vi "Lab Panel V2.4.vi"() -> ()   [LabVIEW 2013]
uses:
  <vilib>/Platform/TimedLoop/XDataNode/timing_clust.ctl
  <vilib>/Platform/TimedLoop/XDataNode/nitl_modes.ctl
  <vilib>/Platform/TimedLoop/XDataNode/wakeup.ctl
  <vilib>/platform/TimedLoop/XDataNode/XDataNode.xnode
  <vilib>/Platform/TimedLoop/XDataNode/XDNodeRunTimeDep.lvlib
panel:
  out "TEMP update":bool
  out "AI update":bool
  in  "stop":bool
  in  "Tab Control 2":T1(tab)
  out "LAB05-2 (SIG)":T2 {"PF" format="%.2f"; "AMPS" format="%.1f"}
  out "LAB05-1 (SIG)":T2 {"PF" format="%.2f"; "AMPS" format="%.1f"}
  out "LAB04-2 (SIG)":T2 {"PF" format="%.2f"; "AMPS" format="%.1f"}
  out "LAB04-1 (SIG)":T2 {"PF" format="%.2f"; "AMPS" format="%.1f"}
  out "LAB03-2 (SIG)":T2 {"PF" format="%.2f"; "AMPS" format="%.1f"}
  out "LAB03-1 (SIG)":T2 {"PF" format="%.2f"; "AMPS" format="%.1f"}
  out "LAB02-2 (SIG)":T2 {"PF" format="%.2f"; "AMPS" format="%.1f"}
  in  "LAB01-1RUN":bool
  in  "LAB05-1 (O/I)":bool
  in  "LAB05-2 (O/I)":bool
  in  "LAB04-1 (O/I)":bool
  in  "LAB04-2 (O/I)":bool
  in  "LAB02-1 (O/I)":bool
  in  "LAB02-2 (O/I)":bool
  in  "LAB01-2 (O/I)":bool
  in  "LAB01-1 (O/I)":bool
  in  "LAB03-1 (O/I)":bool
  in  "LAB05-2 RUN":bool
  in  "LAB05-1 RUN":bool
  in  "LAB04-2 RUN":bool
  in  "LAB04-1 RUN":bool
  in  "LAB03-2 RUN":bool
  in  "LAB03-1 RUN":bool
  in  "LAB02-2 RUN":bool
  in  "LAB02-1 RUN":bool
  in  "LAB01-2 RUN":bool
  in  "LAB05-2 SELECT":T3(radio)
  in  "LAB05-1 SELECT":T3(radio)
  in  "LAB04-2 SELECT":T3(radio)
  in  "LAB04-1 SELECT":T3(radio)
  in  "LAB03-2 SELECT":T3(radio)
  in  "LAB03-1 SELECT":T3(radio)
  in  "LAB02-2 SELECT":T3(radio)
  in  "LAB02-1 SELECT":T3(radio)
  in  "LAB01-2 SELECT":T3(radio)
  in  "LAB01-1 SELECT":T3(radio)
  in  "LAB03-2 (O/I)":bool
  out "LAB01-1 (SIG)":T2 {"PF" format="%.2f"; "AMPS" format="%.1f"}
  out "LAB01-2 (SIG)":T2 {"PF" format="%.2f"; "AMPS" format="%.1f"}
  out "LAB02-1 (SIG)":T2 {"PF" format="%.2f"; "AMPS" format="%.1f"}
  out "LAB05-2 (RESULT)":bool
  out "LAB05-1 (RESULT)":bool
  out "LAB04-2 (RESULT)":bool
  out "LAB04-1 (RESULT)":bool
  out "LAB03-2 (RESULT)":bool
  out "LAB03-1 (RESULT)":bool
  out "LAB02-2 (RESULT)":bool
  out "LAB02-1 (RESULT)":bool
  out "LAB01-2 (RESULT)":bool
  out "LAB01-1 (RESULT)":bool
  in  "LAB05 (SETTINGS 1)":T4={"1 Name"="", "1 Description"="", "1 (CYCLES)"=1.0, "1 (T-RISE mins)"=1.0, "1 (T-RISE deg C)"=1.0, "2 Name"="", "2 Description"="", "2 (CYCLES)"=1.0, "2 (T-RISE mins)"=1.0, "2 (T-RISE deg C)"=1.0} {"2 (T-RISE deg C)" min=1.0 max=100.0 step=1.0 format="%#.0f"; "2 (T-RISE mins)" min=0.0 max=1000.0 step=10.0 format="%#.0f"; "2 (CYCLES)" min=0.0 max=100000.0 step=10.0; "1 (T-RISE deg C)" min=1.0 max=100.0 step=1.0 format="%#.0f"; "1 (T-RISE mins)" min=0.0 max=1000.0 step=10.0 format="%#.0f"; "1 (CYCLES)" min=0.0 max=100000.0 step=10.0}
  in  "LAB04 (SETTINGS 1)":T4={"1 Name"="", "1 Description"="", "1 (CYCLES)"=1.0, "1 (T-RISE mins)"=1.0, "1 (T-RISE deg C)"=1.0, "2 Name"="", "2 Description"="", "2 (CYCLES)"=1.0, "2 (T-RISE mins)"=1.0, "2 (T-RISE deg C)"=1.0} {"2 (T-RISE deg C)" min=1.0 max=100.0 step=1.0 format="%#.0f"; "2 (T-RISE mins)" min=0.0 max=1000.0 step=10.0 format="%#.0f"; "2 (CYCLES)" min=0.0 max=100000.0 step=10.0; "1 (T-RISE deg C)" min=1.0 max=100.0 step=1.0 format="%#.0f"; "1 (T-RISE mins)" min=0.0 max=1000.0 step=10.0 format="%#.0f"; "1 (CYCLES)" min=0.0 max=100000.0 step=10.0}
  in  "LAB03 (SETTINGS 1)":T4={"1 Name"="", "1 Description"="", "1 (CYCLES)"=1.0, "1 (T-RISE mins)"=1.0, "1 (T-RISE deg C)"=1.0, "2 Name"="", "2 Description"="", "2 (CYCLES)"=1.0, "2 (T-RISE mins)"=1.0, "2 (T-RISE deg C)"=1.0} {"2 (T-RISE deg C)" min=1.0 max=100.0 step=1.0 format="%#.0f"; "2 (T-RISE mins)" min=0.0 max=1000.0 step=10.0 format="%#.0f"; "2 (CYCLES)" min=0.0 max=100000.0 step=10.0; "1 (T-RISE deg C)" min=1.0 max=100.0 step=1.0 format="%#.0f"; "1 (T-RISE mins)" min=0.0 max=1000.0 step=10.0 format="%#.0f"; "1 (CYCLES)" min=0.0 max=100000.0 step=10.0}
  out "LAB05 (DISP 1)":T5 {"2 (T-RISE min)" format="%#.0f"; "2 (CYCLE)" format="%#.0f"; "1 (T-RISE min)" format="%#.0f"; "1 (CYCLE)" format="%#.0f"}
  out "LAB04 (DISP 1)":T5 {"2 (T-RISE min)" format="%#.0f"; "2 (CYCLE)" format="%#.0f"; "1 (T-RISE min)" format="%#.0f"; "1 (CYCLE)" format="%#.0f"}
  out "LAB03 (DISP 1)":T5 {"2 (T-RISE min)" format="%#.0f"; "2 (CYCLE)" format="%#.0f"; "1 (T-RISE min)" format="%#.0f"; "1 (CYCLE)" format="%#.0f"}
  out "LAB02 (DISP 1)":T5 {"2 (T-RISE min)" format="%#.0f"; "2 (CYCLE)" format="%#.0f"; "1 (T-RISE min)" format="%#.0f"; "1 (CYCLE)" format="%#.0f"}
  in  "LAB02 (SETTINGS 1)":T4={"1 Name"="", "1 Description"="", "1 (CYCLES)"=1.0, "1 (T-RISE mins)"=1.0, "1 (T-RISE deg C)"=1.0, "2 Name"="", "2 Description"="", "2 (CYCLES)"=1.0, "2 (T-RISE mins)"=1.0, "2 (T-RISE deg C)"=1.0} {"2 (T-RISE deg C)" min=1.0 max=100.0 step=1.0 format="%#.0f"; "2 (T-RISE mins)" min=0.0 max=1000.0 step=10.0 format="%#.0f"; "2 (CYCLES)" min=0.0 max=100000.0 step=10.0; "1 (T-RISE deg C)" min=1.0 max=100.0 step=1.0 format="%#.0f"; "1 (T-RISE mins)" min=0.0 max=1000.0 step=10.0 format="%#.0f"; "1 (CYCLES)" min=0.0 max=100000.0 step=10.0}
  out "LAB01 (DISP 1)":T5 {"2 (T-RISE min)" format="%#.0f"; "2 (CYCLE)" format="%#.0f"; "1 (T-RISE min)" format="%.2f"; "1 (CYCLE)" format="%#.0f"}
  in  "LAB01 (SETTINGS 1)":T4={"1 Name"="", "1 Description"="", "1 (CYCLES)"=1.0, "1 (T-RISE mins)"=1.0, "1 (T-RISE deg C)"=1.0, "2 Name"="", "2 Description"="", "2 (CYCLES)"=1.0, "2 (T-RISE mins)"=1.0, "2 (T-RISE deg C)"=1.0} {"2 (T-RISE deg C)" min=1.0 max=100.0 step=1.0 format="%#.0f"; "2 (T-RISE mins)" min=0.0 max=1000.0 step=10.0 format="%#.0f"; "2 (CYCLES)" min=0.0 max=100000.0 step=10.0; "1 (T-RISE deg C)" min=1.0 max=100.0 step=1.0 format="%#.0f"; "1 (T-RISE mins)" min=1.0 max=1000.0 step=10.0 format="%#.0f"; "1 (CYCLES)" min=1.0 max=100000.0 step=10.0}
  out "LAB05 (TEMP START)":T6
  out "LAB04 (TEMP START)":T6
  out "LAB03 (TEMP START)":T6
  out "LAB02 (TEMP START)":T6
  out "LAB01 (TEMP START)":T6
  in  "JIG ON TIME (S)":dbl=1.0 min=1.0 max=10.0 step=0.5 format="%.1g"
  in  "JIG OFF TIME (S)":dbl=2.0 min=2.0 max=10.0 step=0.5 format="%.1g"
  out "LAB01-1 (JIG)":bool
  out "LAB01-2 (JIG)":bool
  out "LAB02-1 (JIG)":bool
  out "LAB02-2 (JIG)":bool
  out "LAB03-1 (JIG)":bool
  out "LAB03-2 (JIG)":bool
  out "LAB04-1 (JIG)":bool
  out "LAB04-2 (JIG)":bool
  out "LAB05-1 (JIG)":bool
  out "LAB05-2 (JIG)":bool
  out "LAB01 (CAL)":T7 {"2 (TN) cal" min=0.0 step=0.01 format="%.2f"; "2 (TL) cal" min=0.0 step=0.01 format="%.2f"; "2 (PF) cal" min=0.0 step=0.01 format="%.2f"; "2 (V) cal" min=0.0 step=0.01 format="%.2f"; "2 (A) cal" min=0.0 step=0.01 format="%.2f"; "1 (TN) cal" min=0.0 step=0.01 format="%.2f"; "1 (TL) cal" min=0.0 step=0.01 format="%.2f"; "1 (PF) cal" min=0.0 step=0.01 format="%.2f"; "1 (V) cal" min=0.0 step=0.01 format="%.2f"; "1  (A) cal" min=0.0 step=0.01 format="%.2f"}
  out "LAB03 (CAL)":T7 {"2 (TN) cal" min=0.0 step=0.01 format="%.2f"; "2 (TL) cal" min=0.0 step=0.01 format="%.2f"; "2 (PF) cal" min=0.0 step=0.01 format="%.2f"; "2 (V) cal" min=0.0 step=0.01 format="%.2f"; "2 (A) cal" min=0.0 step=0.01 format="%.2f"; "1 (TN) cal" min=0.0 step=0.01 format="%.2f"; "1 (TL) cal" min=0.0 step=0.01 format="%.2f"; "1 (PF) cal" min=0.0 step=0.01 format="%.2f"; "1 (V) cal" min=0.0 step=0.01 format="%.2f"; "1  (A) cal" min=0.0 step=0.01 format="%.2f"}
  out "LAB02 (CAL)":T8 {"2 (TN) cal" min=0.0 step=0.01 format="%.2f"; "2 (TL) cal" min=0.0 step=0.01 format="%.2f"; "2 (PF) cal" min=0.0 step=0.01 format="%.2f"; "2 (V) cal" min=0.0 step=0.01 format="%.2f"; "2 (A) cal" min=0.0 step=0.01 format="%.2f"; "1 (TN) cal" min=0.0 step=0.01 format="%.2f"; "1 (TL) cal" min=0.0 step=0.01 format="%.2f"; "1 (PF) cal" min=0.0 step=0.01 format="%.2f"; "1 (V) cal" min=0.0 step=0.01 format="%.2f"; "1 (A) cal" min=0.0 step=0.01 format="%.2f"}
  out "LAB05 (CAL)":T7 {"2 (TN) cal" min=0.0 step=0.01 format="%.2f"; "2 (TL) cal" min=0.0 step=0.01 format="%.2f"; "2 (PF) cal" min=0.0 step=0.01 format="%.2f"; "2 (V) cal" min=0.0 step=0.01 format="%.2f"; "2 (A) cal" min=0.0 step=0.01 format="%.2f"; "1 (TN) cal" min=0.0 step=0.01 format="%.2f"; "1 (TL) cal" min=0.0 step=0.01 format="%.2f"; "1 (PF) cal" min=0.0 step=0.01 format="%.2f"; "1 (V) cal" min=0.0 step=0.01 format="%.2f"; "1  (A) cal" min=0.0 step=0.01 format="%.2f"}
  out "LAB04 (CAL)":T7 {"2 (TN) cal" min=0.0 step=0.01 format="%.2f"; "2 (TL) cal" min=0.0 step=0.01 format="%.2f"; "2 (PF) cal" min=0.0 step=0.01 format="%.2f"; "2 (V) cal" min=0.0 step=0.01 format="%.2f"; "2 (A) cal" min=0.0 step=0.01 format="%.2f"; "1 (TN) cal" min=0.0 step=0.01 format="%.2f"; "1 (TL) cal" min=0.0 step=0.01 format="%.2f"; "1 (PF) cal" min=0.0 step=0.01 format="%.2f"; "1 (V) cal" min=0.0 step=0.01 format="%.2f"; "1  (A) cal" min=0.0 step=0.01 format="%.2f"}
  out "calibration file error out":errorcluster
  in  "CALIBRATE":bool
  in  "Tab Control":T9(tab)
  out "LAB01-2 (GRAPH)":dynamicdata(graph)
  out "LAB01-1 (GRAPH)":dynamicdata(graph)
  out "LAB02-2 (GRAPH)":dynamicdata(graph)
  out "LAB02-1 (GRAPH)":dynamicdata(graph)
  out "LAB03-2 (GRAPH)":dynamicdata(graph)
  out "LAB03-1 (GRAPH)":dynamicdata(graph)
  out "LAB04-2 (GRAPH)":dynamicdata(graph)
  out "LAB04-1 (GRAPH)":dynamicdata(graph)
  out "LAB05-2 (GRAPH)":dynamicdata(graph)
  out "LAB05-1 (GRAPH)":dynamicdata(graph)
  out "LAB05 TEMP":T10
  out "LAB04 TEMP":T10
  out "LAB02 TEMP":T10
  out "LAB01 TEMP":T10
  out "LAB03 TEMP":T10
  out "Analog Error Array":errorcluster[](array[cluster])
  out "AI loop time":dbl format="%.6g"
  out "loops":dbl
  in  "loop  delay(mS)":dbl
  out "on loops":dbl
  out "off loops":dbl
  out "jig cycle":dbl
  out "LAB01-1 (TDMS)":refnum<k34>
  out "LAB01-2 (TDMS)":refnum<k34>
  out "data file error":errorcluster
  # "LAB01"
  # "LAB02"
  # "LAB05"
  # "LAB03"
  # "LAB04"
  # "LAB01"
  # "LAB02"
  # "LAB03"
  # "LAB04"
  # "LAB05"
  # "JIG SET"
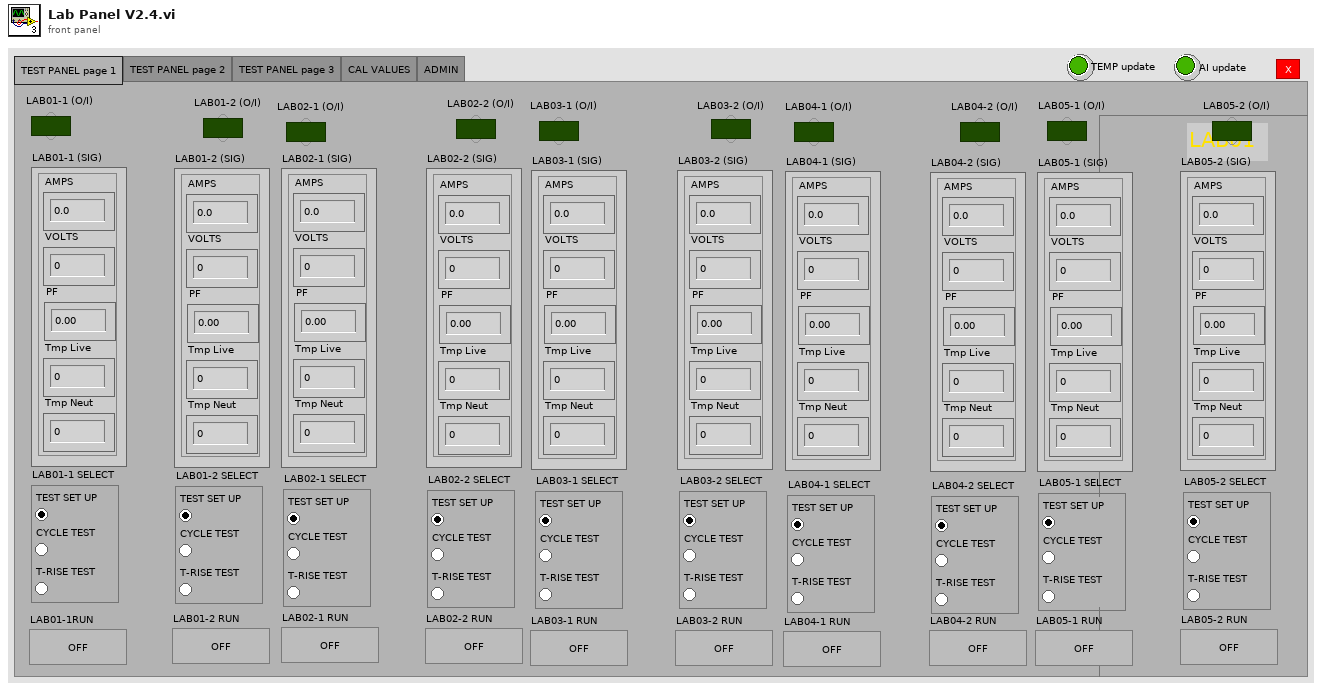
[diagram p1: front panel]
types:
  T1 = enum32{"TEST PANEL page 1", "TEST PANEL page 2", "TEST PANEL page 3", "CAL VALUES", "ADMIN"}
  T2 = cluster{"AMPS":dbl, "VOLTS":dbl, "PF":dbl, "Tmp Live":dbl, "Tmp Neut":dbl}
  T3 = enum32{"TEST SET UP", "CYCLE TEST", "T-RISE TEST"}
  T4 = cluster{"1 Name":string, "1 Description":string, "1 (CYCLES)":dbl, "1 (T-RISE mins)":dbl, "1 (T-RISE deg C)":dbl, "2 Name":string, "2 Description":string, "2 (CYCLES)":dbl, "2 (T-RISE mins)":dbl, "2 (T-RISE deg C)":dbl}
  T5 = cluster{"1 (CYCLE)":dbl, "1 (T-RISE min)":dbl, "1 (STATUS)":string, "2 (CYCLE)":dbl, "2 (T-RISE min)":dbl, "2 (STATUS)":string}
  T6 = cluster{"1 (TL)":dbl, "1 (TN)":dbl, "2 (TL)":dbl, "2 (TN)":dbl}
  T7 = cluster{"1  (A) cal":dbl, "1 (V) cal":dbl, "1 (PF) cal":dbl, "1 (TL) cal":dbl, "1 (TN) cal":dbl, "2 (A) cal":dbl, "2 (V) cal":dbl, "2 (PF) cal":dbl, "2 (TL) cal":dbl, "2 (TN) cal":dbl}
  T8 = cluster{"1 (A) cal":dbl, "1 (V) cal":dbl, "1 (PF) cal":dbl, "1 (TL) cal":dbl, "1 (TN) cal":dbl, "2 (A) cal":dbl, "2 (V) cal":dbl, "2 (PF) cal":dbl, "2 (TL) cal":dbl, "2 (TN) cal":dbl}
  T9 = enum32{"LAB01", "LAB02", "LAB03", "LAB04", "LAB05", "TEMPERATURE", "ERROR"}
  T10 = cluster{"T1 Live":dbl, "T1 Neut":dbl, "T2 Live":dbl, "T2 Neut":dbl, "ID":dbl, "ER":dbl}
  T11 = typedef "XDNodeRunTimeDep.lvlib/timing_clust.ctl" = cluster{"Expected End [f-1]":u64, "Actual End [f-1]":u64, "Finished Late? [f-1]":bool, "Expected End [i-1]":u64, "Actual End [i-1]":u64, "Finished Late? [i-1]":bool, "Expected Start [i]":u64, "Actual Start [i]":u64, "Expected Start [f]":u64, "Actual Start [f]":u64, "Source Name":string, "Structure Name":string, "Period":i64, "Deadline":i64, "Offset":i64, "Start":i64, "Priority":i32, "Timeout":i32, "Mode":T12, "Wakeup Reason":T13, "Error":errorcluster, "Source Type":string, "Secondary Source Type":string, "Global End Time":u64, "Global Start Time":u64, "Frame Duration":u64, "Iteration Duration":u64, "Assigned CPU":i32, "I/O Scan Engine Mode":u32}
  T12 = typedef "XDNodeRunTimeDep.lvlib/nitl_modes.ctl" = enum32{"No Change", "Process missed periods, maintain original phase", "Discard missed periods, maintain original phase", "Process missed periods, ignore original phase", "Discard missed periods, ignore original phase"}
  T13 = typedef "XDNodeRunTimeDep.lvlib/wakeup.ctl" = enum32{"Normal", "Aborted", "Asynchronous wakeup", "Timing source error", "Timed loop error", "Timeout"}
  T14 = enum16{"open", "open or create", "create or replace", "create", "open (read-only)"}
  T15 = cluster{"T1":dbl, "T2":dbl, "T3":dbl, "T4":dbl, "ID":dbl, "ER":dbl}
  T16 = cluster{"LAB01-1 (A)":dbl, "LAB01-1 (V)":dbl, "LAB01-1 (PF)":dbl, "LAB01-2 (A)":dbl, "LAB01-2 (V)":dbl, "LAB01-2 (PF)":dbl}
  T17 = cluster{"LAB02-1 (A)":dbl, "LAB02-1 (V)":dbl, "LAB02-1 (PF)":dbl, "LAB02-2 (A)":dbl, "LAB02-2 (V)":dbl, "LAB02-2 (PF)":dbl}
  T18 = cluster{"LAB03-1 (A)":dbl, "LAB03-1 (V)":dbl, "LAB03-1 (PF)":dbl, "LAB03-2 (A)":dbl, "LAB03-2 (V)":dbl, "LAB03-2 (PF)":dbl}
  T19 = cluster{"LAB04-1 (A)":dbl, "LAB04-1 (V)":dbl, "LAB04-1 (PF)":dbl, "LAB04-2 (A)":dbl, "LAB04-2 (V)":dbl, "LAB04-2 (PF)":dbl}
  T20 = cluster{"LAB05-1 (A)":dbl, "LAB05-1 (V)":dbl, "LAB05-1 (PF)":dbl, "LAB05-2 (A)":dbl, "LAB05-2 (V)":dbl, "LAB05-2 (PF)":dbl}
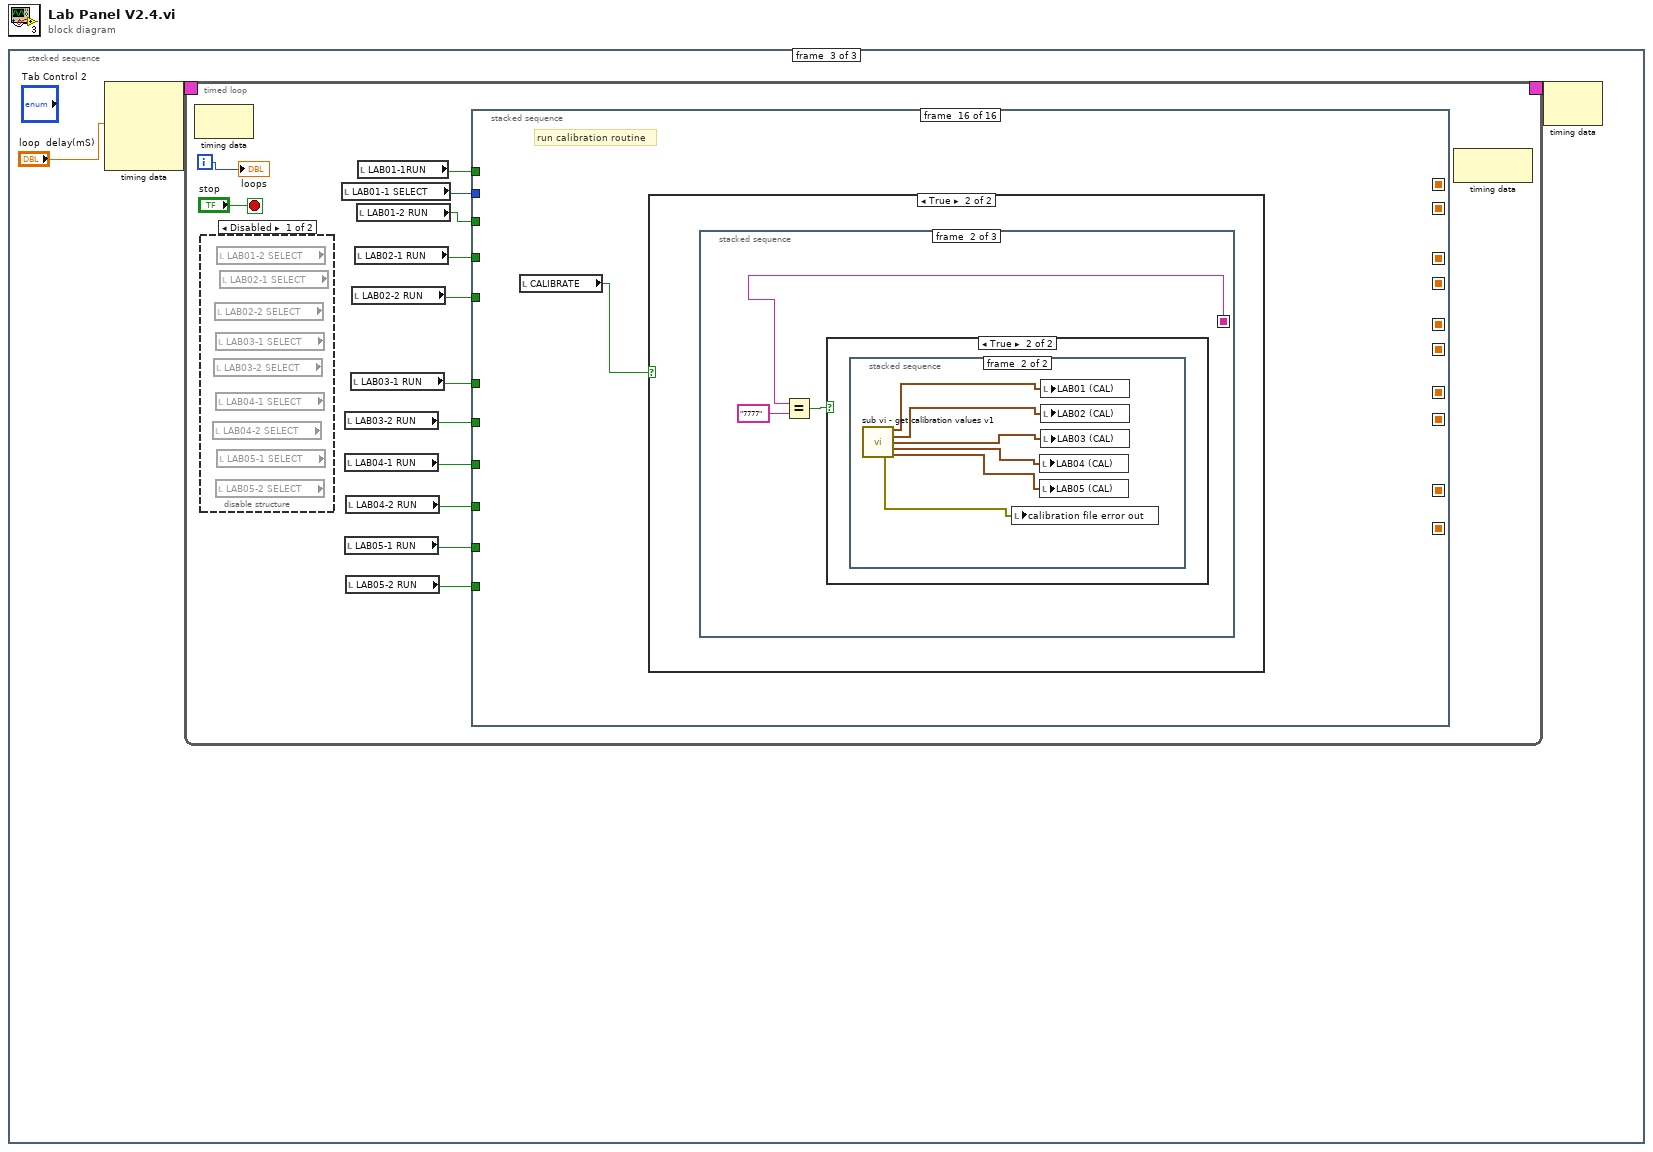
[diagram p0: block diagram]
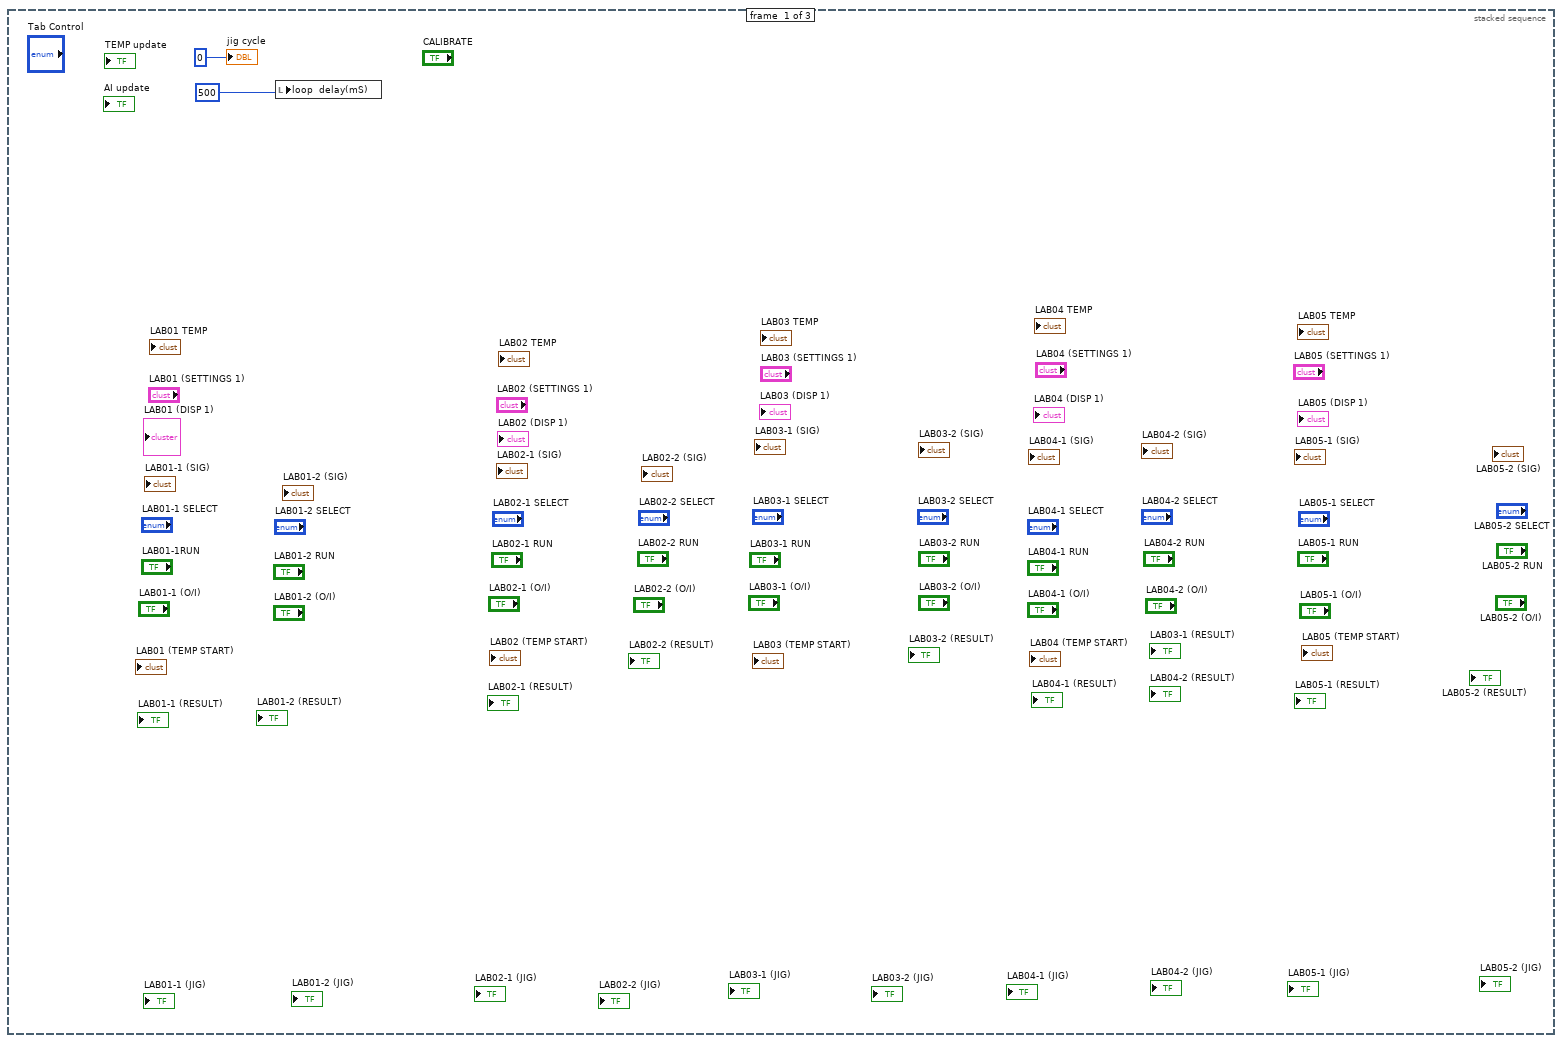
[diagram p2: hidden frame]
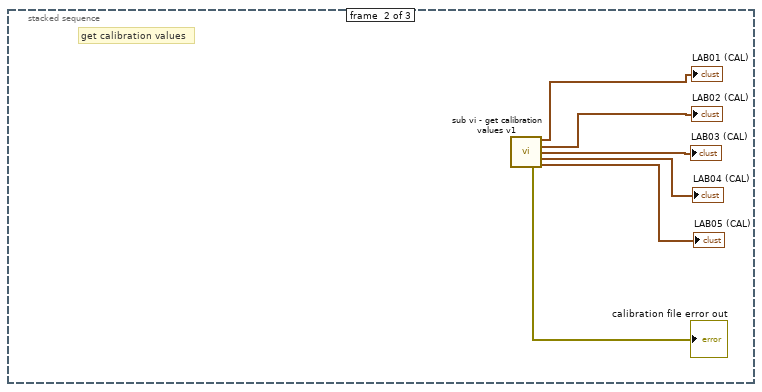
[diagram p3: hidden frame]
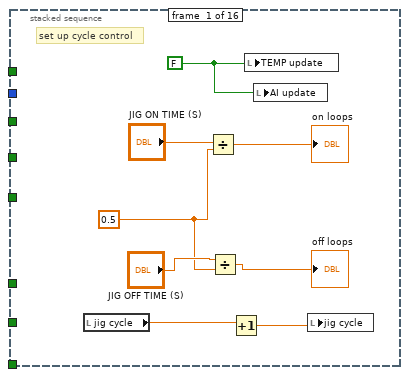
[diagram p5: hidden frame]
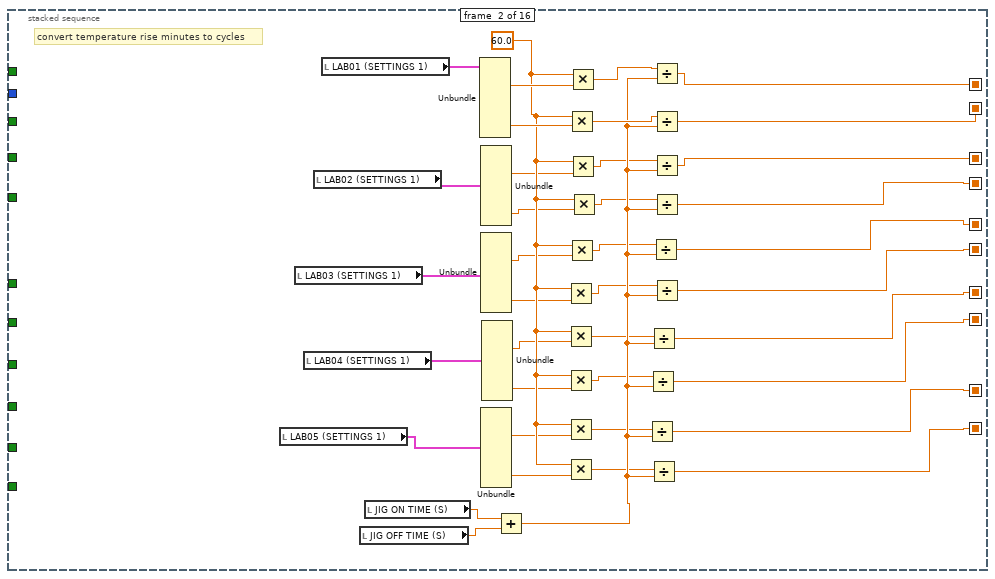
[diagram p6: hidden frame]
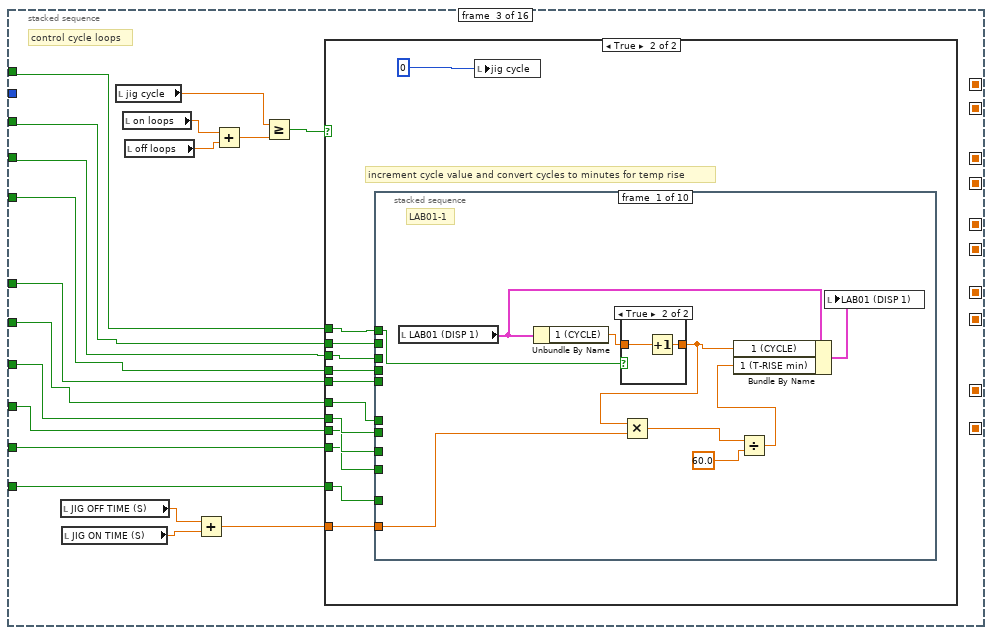
[diagram p7: hidden frame]
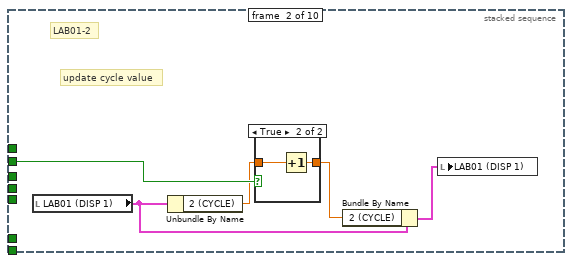
[diagram p10: hidden frame]
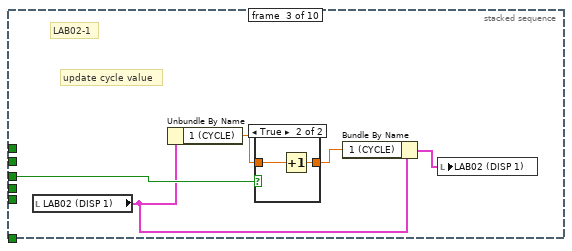
[diagram p12: hidden frame]
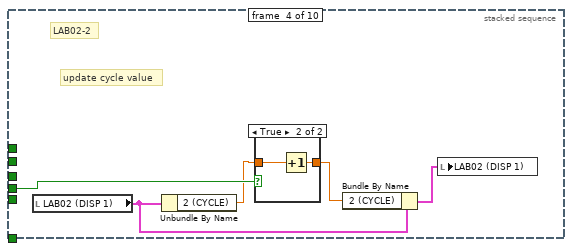
[diagram p14: hidden frame]
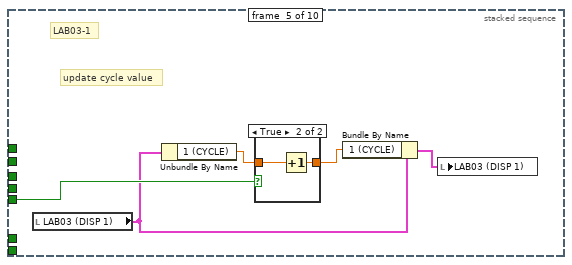
[diagram p16: hidden frame]
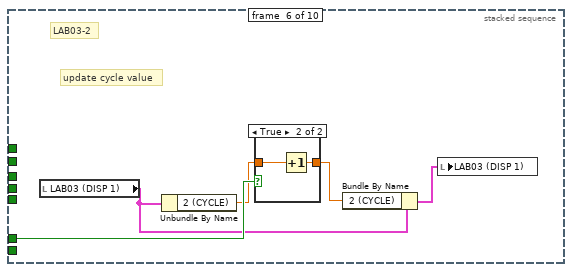
[diagram p18: hidden frame]
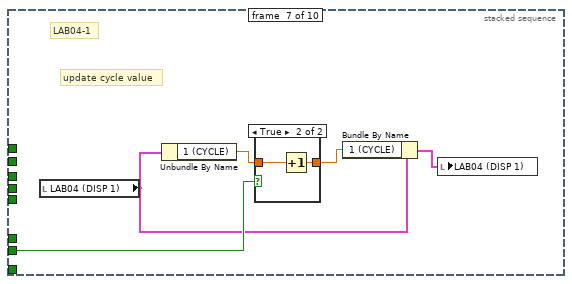
[diagram p20: hidden frame]
diagram:
  n1 = stacked-sequence {
    frame #0 {
      n2 = local write "loop  delay(mS)"(500) -> ()
      "jig cycle" <- 0
    }
    frame #1 {
      # "get calibration values"
      n3 = call "sub vi - get calibration values v1.vi"() -> ("LAB01 (CAL)"=→"LAB01 (CAL)":T7, "LAB02 (CAL)"=→"LAB02 (CAL)":T8, "LAB03 (CAL)"=→"LAB03 (CAL)":T7, "LAB04 (CAL)"=→"LAB04 (CAL)":T7, "calibration file error out"=→"calibration file error out":errorcluster, "LAB05 (CAL)"=→"LAB05 (CAL)":T7)  [unwired: 10 in]
    }
    frame #2 {
      n4 = node-c288("loop  delay(mS)") -> (w11:T11)  [unwired: 3 in]
      n5 = timed-loop {
        timing: w11 -> [_]
        timing-out: [_] -> w10
        i -> [w24]
        stop <- "stop" stop-if-true
        n6 = node-c288() -> ()  [unwired: 1 in, 1 out]
        n7 = disable-structure shown="Disabled" {
          frame Disabled {
            n8 = local read "LAB04-2 SELECT"() -> ()  [unwired: 1 out]
            n9 = local read "LAB03-2 SELECT"() -> ()  [unwired: 1 out]
            n10 = local read "LAB02-2 SELECT"() -> ()  [unwired: 1 out]
            n11 = local read "LAB03-1 SELECT"() -> ()  [unwired: 1 out]
            n12 = local read "LAB04-1 SELECT"() -> ()  [unwired: 1 out]
            n13 = local read "LAB05-2 SELECT"() -> ()  [unwired: 1 out]
            n14 = local read "LAB01-2 SELECT"() -> ()  [unwired: 1 out]
            n15 = local read "LAB05-1 SELECT"() -> ()  [unwired: 1 out]
            n16 = local read "LAB02-1 SELECT"() -> ()  [unwired: 1 out]
          }
          frame Enabled {
          }
        }
        n17 = local read "LAB01-1 SELECT"() -> (w12:T3)
        n18 = local read "LAB03-2 RUN"() -> (w17:bool)
        n19 = local read "LAB04-1 RUN"() -> (w16:bool)
        n20 = local read "LAB05-1 RUN"() -> (w14:bool)
        n21 = local read "LAB04-2 RUN"() -> (w15:bool)
        n22 = local read "LAB05-2 RUN"() -> (w13:bool)
        n23 = local read "LAB03-1 RUN"() -> (w18:bool)
        n24 = local read "LAB02-2 RUN"() -> (w19:bool)
        n25 = local read "LAB02-1 RUN"() -> (w20:bool)
        n26 = local read "LAB01-2 RUN"() -> (w21:bool)
        n27 = local read "LAB01-1RUN"() -> (w22:bool)
        n28 = stacked-sequence {
          seq-local: [_ w70 _ _ _ _ _ _ _ _ _ _ _ _ _ _] -> [_ _ _ _ w235 _ _ _ _ _ _ _ _ _ _ _]
          seq-local: [_ w69 _ _ _ _ _ _ _ _ _ _ _ _ _ _] -> [_ _ _ _ _ _ _ _ _ _ _ _ _ _ _ _]
          seq-local: [_ w42 _ _ _ _ _ _ _ _ _ _ _ _ _ _] -> [_ _ _ _ _ _ _ _ _ _ _ _ _ _ _ _]
          seq-local: [_ w41 _ _ _ _ _ _ _ _ _ _ _ _ _ _] -> [_ _ _ _ _ _ _ _ _ _ _ _ _ _ _ _]
          seq-local: [_ w40 _ _ _ _ _ _ _ _ _ _ _ _ _ _] -> [_ _ _ _ _ _ _ _ _ _ _ _ _ _ _ _]
          seq-local: [_ w39 _ _ _ _ _ _ _ _ _ _ _ _ _ _] -> [_ _ _ _ _ _ _ _ _ _ _ _ _ _ _ _]
          seq-local: [_ w38 _ _ _ _ _ _ _ _ _ _ _ _ _ _] -> [_ _ _ _ _ _ _ _ _ _ _ _ _ _ _ _]
          seq-local: [_ w37 _ _ _ _ _ _ _ _ _ _ _ _ _ _] -> [_ _ _ _ _ _ _ _ _ _ _ _ _ _ _ _]
          seq-local: [_ w36 _ _ _ _ _ _ _ _ _ _ _ _ _ _] -> [_ _ _ _ _ _ _ _ _ _ _ _ _ _ _ _]
          seq-local: [_ w35 _ _ _ _ _ _ _ _ _ _ _ _ _ _] -> [_ _ _ _ _ _ _ _ _ _ _ _ _ _ _ _]
          tunnel: w22 -> [_ _ w87 w198 w246 w283 w346 _ _ _ _ _ w809 w865 w924 _]
          tunnel: w21 -> [_ _ w86 w197 w245 w282 _ _ _ _ _ _ _ _ _ _]
          tunnel: w20 -> [_ _ w85 w196 w244 w281 _ _ _ _ _ _ _ _ _ _]
          tunnel: w19 -> [_ _ w84 w195 w243 w280 _ _ _ _ _ _ _ _ _ _]
          tunnel: w18 -> [_ _ w83 w194 w242 w279 _ _ _ _ _ _ _ _ _ _]
          tunnel: w17 -> [_ _ w82 w193 w241 w278 _ _ _ _ _ _ _ _ _ _]
          tunnel: w16 -> [_ _ w81 w192 w240 w277 _ _ _ _ _ _ _ _ _ _]
          tunnel: w15 -> [_ _ w80 w191 w239 w276 _ _ _ _ _ _ _ _ _ _]
          tunnel: w14 -> [_ _ w79 w190 w238 w275 _ _ _ _ _ _ _ _ _ _]
          tunnel: w13 -> [_ _ w78 w189 w237 w274 _ _ _ _ _ _ _ _ _ _]
          tunnel: w12 -> [_ _ _ w188 w236 _ w347 _ _ _ _ _ _ w867 w925 _]
          frame #0 {
            w27 = FALSE
            w32 = 0.5
            # "set up cycle control"
            n29 = local read "jig cycle"() -> (w31:dbl)
            n30 = Divide(x="JIG ON TIME (S)", y=w32) -> (x/y=→"on loops":dbl)
            n31 = Divide(x="JIG OFF TIME (S)", y=w32) -> (x/y=→"off loops":dbl)
            n32 = Increment(x=w31) -> (x+1=w30:dbl)
            n33 = local write "TEMP update"(w27) -> ()
            n34 = local write "AI update"(w27) -> ()
            n35 = local write "jig cycle"(w30) -> ()
          }
          frame #1 {
            w60 = 60.0
            # "convert temperature rise minutes to cycles"
            n36 = local read "LAB05 (SETTINGS 1)"() -> (w61:T4)
            n37 = local read "LAB03 (SETTINGS 1)"() -> (w63:T4)
            n38 = local read "LAB04 (SETTINGS 1)"() -> (w62:T4)
            n39 = local read "LAB02 (SETTINGS 1)"() -> (w64:T4)
            n40 = local read "LAB01 (SETTINGS 1)"() -> (w73:T4)
            n41 = local read "JIG OFF TIME (S)"() -> (w71:dbl)
            n42 = local read "JIG ON TIME (S)"() -> (w72:dbl)
            n43 = Unbundle(w73) -> ("1 (T-RISE mins)"=w68:dbl, "2 (T-RISE mins)"=w67:dbl)  [unwired: 8 out]
            n44 = Unbundle(w64) -> ("1 (T-RISE mins)"=w59:dbl, "2 (T-RISE mins)"=w58:dbl)  [unwired: 8 out]
            n45 = Unbundle(w63) -> ("1 (T-RISE mins)"=w57:dbl, "2 (T-RISE mins)"=w56:dbl)  [unwired: 8 out]
            n46 = Unbundle(w61) -> ("1 (T-RISE mins)"=w53:dbl, "2 (T-RISE mins)"=w52:dbl)  [unwired: 8 out]
            n47 = Unbundle(w62) -> ("1 (T-RISE mins)"=w55:dbl, "2 (T-RISE mins)"=w54:dbl)  [unwired: 8 out]
            n48 = Add(x=w72, y=w71) -> (x+y=w51:dbl)
            n49 = Multiply(x=w60, y=w56) -> (x*y=w47:dbl)
            n50 = Multiply(x=w60, y=w55) -> (x*y=w46:dbl)
            n51 = Multiply(x=w60, y=w54) -> (x*y=w45:dbl)
            n52 = Multiply(x=w60, y=w53) -> (x*y=w44:dbl)
            n53 = Multiply(x=w60, y=w52) -> (x*y=w43:dbl)
            n54 = Multiply(x=w60, y=w67) -> (x*y=w65:dbl)
            n55 = Multiply(x=w60, y=w57) -> (x*y=w48:dbl)
            n56 = Multiply(x=w60, y=w68) -> (x*y=w66:dbl)
            n57 = Multiply(x=w60, y=w59) -> (x*y=w50:dbl)
            n58 = Multiply(x=w60, y=w58) -> (x*y=w49:dbl)
            n59 = Divide(x=w44, y=w51) -> (x/y=w36:dbl)
            n60 = Divide(x=w45, y=w51) -> (x/y=w37:dbl)
            n61 = Divide(x=w46, y=w51) -> (x/y=w38:dbl)
            n62 = Divide(x=w43, y=w51) -> (x/y=w35:dbl)
            n63 = Divide(x=w48, y=w51) -> (x/y=w40:dbl)
            n64 = Divide(x=w66, y=w51) -> (x/y=w70:dbl)
            n65 = Divide(x=w65, y=w51) -> (x/y=w69:dbl)
            n66 = Divide(x=w50, y=w51) -> (x/y=w42:dbl)
            n67 = Divide(x=w49, y=w51) -> (x/y=w41:dbl)
            n68 = Divide(x=w47, y=w51) -> (x/y=w39:dbl)
          }
          frame #2 {
            # "control cycle loops"
            n69 = local read "JIG OFF TIME (S)"() -> (w76:dbl)
            n70 = local read "JIG ON TIME (S)"() -> (w75:dbl)
            n71 = local read "jig cycle"() -> (w89:dbl)
            n72 = local read "on loops"() -> (w91:dbl)
            n73 = local read "off loops"() -> (w90:dbl)
            n74 = Add(x=w76, y=w75) -> (x+y=w74:dbl)
            n75 = Add(x=w91, y=w90) -> (x+y=w77:dbl)
            n76 = Greater Or Equal?(x=w89, y=w77) -> (x >= y?=w88:bool)
            n77 = case shown="True" w88 {
              tunnel: w87 -> [_ w102]
              tunnel: w86 -> [_ w101]
              tunnel: w85 -> [_ w100]
              tunnel: w84 -> [_ w99]
              tunnel: w83 -> [_ w98]
              tunnel: w82 -> [_ w97]
              tunnel: w81 -> [_ w96]
              tunnel: w80 -> [_ w95]
              tunnel: w79 -> [_ w94]
              tunnel: w78 -> [_ w93]
              tunnel: w74 -> [_ w92]
              frame False {
              }
              frame True {
                # "increment cycle value and convert cycles to minutes for temp rise"
                n78 = stacked-sequence {
                  tunnel: w102 -> [w112 _ _ _ _ _ _ _ _ _]
                  tunnel: w101 -> [_ w120 _ _ _ _ _ _ _ _]
                  tunnel: w100 -> [_ _ w128 _ _ _ _ _ _ _]
                  tunnel: w99 -> [_ _ _ w136 _ _ _ _ _ _]
                  tunnel: w98 -> [_ _ _ _ w144 _ _ _ _ _]
                  tunnel: w97 -> [_ _ _ _ _ w152 _ _ _ _]
                  tunnel: w96 -> [_ _ _ _ _ _ w160 _ _ _]
                  tunnel: w95 -> [_ _ _ _ _ _ _ w168 _ _]
                  tunnel: w94 -> [_ _ _ _ _ _ _ _ w176 _]
                  tunnel: w93 -> [_ _ _ _ _ _ _ _ _ w184]
                  tunnel: w92 -> [w104 _ _ _ _ _ _ _ _ _]
                  frame #0 {
                    # "LAB01-1"
                    n79 = local read "LAB01 (DISP 1)"() -> (w109:T5)
                    n80 = Unbundle By Name(w109) -> ("1 (CYCLE)"=w110:dbl)
                    n81 = case shown="True" w112 {
                      tunnel: w110 -> [w113 w115]
                      tunnel: [w113 w114] -> w106
                      frame False {
                      }
                      frame True {
                        n82 = Increment(x=w115) -> (x+1=w114:dbl)
                      }
                    }
                    n83 = Multiply(x=w106, y=w104) -> (x*y=w105:dbl)
                    n84 = Divide(x=w105, y=60.0) -> (x/y=w107:dbl)
                    n85 = Bundle By Name(cluster=w109, "1 (CYCLE)"=w106, "1 (T-RISE min)"=w107) -> (w111:T5)
                    n86 = local write "LAB01 (DISP 1)"(w111) -> ()
                  }
                  frame #1 {
                    # "update cycle value"
                    # "LAB01-2"
                    n87 = local read "LAB01 (DISP 1)"() -> (w118:T5)
                    n88 = Unbundle By Name(w118) -> ("2 (CYCLE)"=w117:dbl)
                    n89 = case shown="True" w120 {
                      tunnel: w117 -> [w121 w123]
                      tunnel: [w121 w122] -> w116
                      frame False {
                      }
                      frame True {
                        n90 = Increment(x=w123) -> (x+1=w122:dbl)
                      }
                    }
                    n91 = Bundle By Name(cluster=w118, "2 (CYCLE)"=w116) -> (w119:T5)
                    n92 = local write "LAB01 (DISP 1)"(w119) -> ()
                  }
                  frame #2 {
                    # "update cycle value"
                    # "LAB02-1"
                    n93 = local read "LAB02 (DISP 1)"() -> (w126:T5)
                    n94 = Unbundle By Name(w126) -> ("1 (CYCLE)"=w124:dbl)
                    n95 = case shown="True" w128 {
                      tunnel: [w129 w131] -> w125
                      tunnel: w124 -> [w129 w130]
                      frame False {
                      }
                      frame True {
                        n96 = Increment(x=w130) -> (x+1=w131:dbl)
                      }
                    }
                    n97 = Bundle By Name(cluster=w126, "1 (CYCLE)"=w125) -> (w127:T5)
                    n98 = local write "LAB02 (DISP 1)"(w127) -> ()
                  }
                  frame #3 {
                    # "update cycle value"
                    # "LAB02-2"
                    n99 = local read "LAB02 (DISP 1)"() -> (w134:T5)
                    n100 = Unbundle By Name(w134) -> ("2 (CYCLE)"=w133:dbl)
                    n101 = case shown="True" w136 {
                      tunnel: [w137 w139] -> w132
                      tunnel: w133 -> [w137 w138]
                      frame False {
                      }
                      frame True {
                        n102 = Increment(x=w138) -> (x+1=w139:dbl)
                      }
                    }
                    n103 = Bundle By Name(cluster=w134, "2 (CYCLE)"=w132) -> (w135:T5)
                    n104 = local write "LAB02 (DISP 1)"(w135) -> ()
                  }
                  frame #4 {
                    # "update cycle value"
                    # "LAB03-1"
                    n105 = local read "LAB03 (DISP 1)"() -> (w142:T5)
                    n106 = Unbundle By Name(w142) -> ("1 (CYCLE)"=w141:dbl)
                    n107 = case shown="True" w144 {
                      tunnel: [w145 w147] -> w140
                      tunnel: w141 -> [w145 w146]
                      frame False {
                      }
                      frame True {
                        n108 = Increment(x=w146) -> (x+1=w147:dbl)
                      }
                    }
                    n109 = Bundle By Name(cluster=w142, "1 (CYCLE)"=w140) -> (w143:T5)
                    n110 = local write "LAB03 (DISP 1)"(w143) -> ()
                  }
                  frame #5 {
                    # "update cycle value"
                    # "LAB03-2"
                    n111 = local read "LAB03 (DISP 1)"() -> (w150:T5)
                    n112 = Unbundle By Name(w150) -> ("2 (CYCLE)"=w149:dbl)
                    n113 = case shown="True" w152 {
                      tunnel: [w153 w155] -> w148
                      tunnel: w149 -> [w153 w154]
                      frame False {
                      }
                      frame True {
                        n114 = Increment(x=w154) -> (x+1=w155:dbl)
                      }
                    }
                    n115 = Bundle By Name(cluster=w150, "2 (CYCLE)"=w148) -> (w151:T5)
                    n116 = local write "LAB03 (DISP 1)"(w151) -> ()
                  }
                  frame #6 {
                    # "update cycle value"
                    # "LAB04-1"
                    n117 = local read "LAB04 (DISP 1)"() -> (w158:T5)
                    n118 = Unbundle By Name(w158) -> ("1 (CYCLE)"=w157:dbl)
                    n119 = case shown="True" w160 {
                      tunnel: [w161 w163] -> w156
                      tunnel: w157 -> [w161 w162]
                      frame False {
                      }
                      frame True {
                        n120 = Increment(x=w162) -> (x+1=w163:dbl)
                      }
                    }
                    n121 = Bundle By Name(cluster=w158, "1 (CYCLE)"=w156) -> (w159:T5)
                    n122 = local write "LAB04 (DISP 1)"(w159) -> ()
                  }
                  frame #7 {
                    # "update cycle value"
                    # "LAB04-2"
                    n123 = local read "LAB04 (DISP 1)"() -> (w166:T5)
                    n124 = Unbundle By Name(w166) -> ("2 (CYCLE)"=w165:dbl)
                    n125 = case shown="True" w168 {
                      tunnel: [w169 w171] -> w164
                      tunnel: w165 -> [w169 w170]
                      frame False {
                      }
                      frame True {
                        n126 = Increment(x=w170) -> (x+1=w171:dbl)
                      }
                    }
                    n127 = Bundle By Name(cluster=w166, "2 (CYCLE)"=w164) -> (w167:T5)
                    n128 = local write "LAB04 (DISP 1)"(w167) -> ()
                  }
                  frame #8 {
                    # "update cycle value"
                    # "LAB05-1"
                    n129 = local read "LAB05 (DISP 1)"() -> (w174:T5)
                    n130 = Unbundle By Name(w174) -> ("1 (CYCLE)"=w173:dbl)
                    n131 = case shown="True" w176 {
                      tunnel: [w177 w179] -> w172
                      tunnel: w173 -> [w177 w178]
                      frame False {
                      }
                      frame True {
                        n132 = Increment(x=w178) -> (x+1=w179:dbl)
                      }
                    }
                    n133 = Bundle By Name(cluster=w174, "1 (CYCLE)"=w172) -> (w175:T5)
                    n134 = local write "LAB05 (DISP 1)"(w175) -> ()
                  }
                  frame #9 {
                    # "update cycle value"
                    # "LAB05-2"
                    n135 = local read "LAB05 (DISP 1)"() -> (w182:T5)
                    n136 = Unbundle By Name(w182) -> ("2 (CYCLE)"=w181:dbl)
                    n137 = case shown="True" w184 {
                      tunnel: [w185 w187] -> w180
                      tunnel: w181 -> [w185 w186]
                      frame False {
                      }
                      frame True {
                        n138 = Increment(x=w186) -> (x+1=w187:dbl)
                      }
                    }
                    n139 = Bundle By Name(cluster=w182, "2 (CYCLE)"=w180) -> (w183:T5)
                    n140 = local write "LAB05 (DISP 1)"(w183) -> ()
                  }
                }
                n141 = local write "jig cycle"(0) -> ()
              }
            }
          }
          frame #3 {
            # "check if test cycles reached for cycle tests, if so then test pass"
            n142 = stacked-sequence {
              tunnel: w198 -> [_]
              tunnel: w197 -> [_]
              tunnel: w196 -> [_]
              tunnel: w195 -> [_]
              tunnel: w194 -> [_]
              tunnel: w193 -> [_]
              tunnel: w192 -> [_]
              tunnel: w191 -> [_]
              tunnel: w190 -> [_]
              tunnel: w189 -> [_]
              tunnel: w188 -> [w203]
              frame #0 {
                # "LAB01-1"
                n143 = Less?(x=w203, y=2) -> (x < y?=w201:bool)
                n144 = local read "LAB01 (DISP 1)"() -> (w204:T5)
                n145 = Unbundle(w204) -> ("1 (STATUS)"=w205:string)  [unwired: 5 out]
                n146 = Equal?(x=w205, y="RUN") -> (x = y?=w200:bool)
                n147 = And(x=w200, y=w201) -> (x .and. y?=w199:bool)
                n148 = case shown="True" w199 {
                  tunnel: w204 -> [_ w212]
                  tunnel: w203 -> [_ w211]
                  frame False {
                  }
                  frame True {
                    n149 = local read "LAB01 (SETTINGS 1)"() -> (w214:T4)
                    n150 = Unbundle(w212) -> ("1 (CYCLE)"=w213:dbl)  [unwired: 5 out]
                    n151 = Unbundle(w214) -> ("1 (CYCLES)"=w208:dbl, "1 (T-RISE mins)"=w210:dbl)  [unwired: 8 out]
                    n152 = case shown="\"TEST SET UP\", Default" w211 {
                      tunnel: w210 -> [_ _ w221]
                      tunnel: [w216 w218 w221] -> w209
                      tunnel: w208 -> [w216 w218 _]
                      tunnel: ["TEST SET UP CYCLES" "CYCLES" "T-RISE TEST"] -> w207
                      frame "TEST SET UP", Default {
                      }
                      frame "CYCLE TEST" {
                      }
                      frame "T-RISE TEST" {
                      }
                    }
                    n153 = Greater Or Equal?(x=w213, y=w208) -> (x >= y?=w215:bool)
                    n154 = case shown="True" w215 {
                      tunnel: w209 -> [w223 _]
                      tunnel: w207 -> [w222 _]
                      frame True {
                        n155 = stacked-sequence {
                          tunnel: w223 -> [w226 _]
                          tunnel: w222 -> [w224 _]
                          frame #0 {
                            n156 = local read "LAB01-1 (TDMS)"() -> (w230:refnum<k34>)
                            n157 = Build Array(w224) -> (w227:string[])
                            n158 = Build Array(w226) -> (w225:dbl[])
                            n159 = TDMS Write(0:w230, 5:"TEST PASS", 7:w227, 9:w225) -> (15:w229:errorcluster)  [unwired: 2 in, 3 out]
                            n160 = local write "data file error"(w229) -> ()
                          }
                          frame #1 {
                            n161 = local read "LAB01 (DISP 1)"() -> (w234:T5)
                            n162 = Bundle(cluster=w234, "1 (STATUS)"="STOP") -> (w232:T5)  [unwired: 5 in]
                            n163 = local write "LAB01-1 (RESULT)"(TRUE) -> ()
                            n164 = local write "LAB01 (DISP 1)"(w232) -> ()
                          }
                        }
                      }
                      frame False {
                      }
                    }
                  }
                }
              }
            }
          }
          frame #4 {
            # "check if test cycles reached for temperature rise test"
            n165 = stacked-sequence {
              tunnel: w246 -> [_]
              tunnel: w245 -> [_]
              tunnel: w244 -> [_]
              tunnel: w243 -> [_]
              tunnel: w242 -> [_]
              tunnel: w241 -> [_]
              tunnel: w240 -> [_]
              tunnel: w239 -> [_]
              tunnel: w238 -> [_]
              tunnel: w237 -> [_]
              tunnel: w236 -> [w252]
              tunnel: w235 -> [w247]
              frame #0 {
                # "LAB01-1"
                n166 = Equal?(x=w252, y=2) -> (x = y?=w250:bool)
                n167 = local read "LAB01 (DISP 1)"() -> (w253:T5)
                n168 = Unbundle(w253) -> ("1 (STATUS)"=w254:string)  [unwired: 5 out]
                n169 = Equal?(x=w254, y="RUN") -> (x = y?=w249:bool)
                n170 = And(x=w249, y=w250) -> (x .and. y?=w248:bool)
                n171 = case shown="True" w248 {
                  tunnel: w253 -> [_ w259]
                  tunnel: w247 -> [_ w258]
                  frame False {
                  }
                  frame True {
                    n172 = local read "LAB01 (SETTINGS 1)"() -> (w257:T4)
                    n173 = Unbundle(w259) -> ("1 (CYCLE)"=w260:dbl)  [unwired: 5 out]
                    n174 = Unbundle(w257) -> ("1 (T-RISE mins)"=w256:dbl)  [unwired: 9 out]
                    n175 = Greater Or Equal?(x=w260, y=w258) -> (x >= y?=w261:bool)
                    n176 = case shown="True" w261 {
                      tunnel: w256 -> [w262 _]
                      frame True {
                        n177 = stacked-sequence {
                          tunnel: w262 -> [w264 _]
                          frame #0 {
                            n178 = local read "LAB01-1 (TDMS)"() -> (w269:refnum<k34>)
                            n179 = Build Array("T-RISE") -> (w266:string[])
                            n180 = Build Array(w264) -> (w265:dbl[])
                            n181 = TDMS Write(0:w269, 5:"TEST PASS", 7:w266, 9:w265) -> (15:w268:errorcluster)  [unwired: 2 in, 3 out]
                            n182 = local write "data file error"(w268) -> ()
                          }
                          frame #1 {
                            n183 = local read "LAB01 (DISP 1)"() -> (w273:T5)
                            n184 = Bundle(cluster=w273, "1 (STATUS)"="STOP") -> (w271:T5)  [unwired: 5 in]
                            n185 = local write "LAB01-1 (RESULT)"(TRUE) -> ()
                            n186 = local write "LAB01 (DISP 1)"(w271) -> ()
                          }
                        }
                      }
                      frame False {
                      }
                    }
                  }
                }
              }
            }
          }
          frame #5 {
            # "disable functions"
            n187 = stacked-sequence {
              tunnel: w283 -> [w293 _ w343]
              tunnel: w282 -> [w292 _ w342]
              tunnel: w281 -> [w291 _ w341]
              tunnel: w280 -> [w290 _ w340]
              tunnel: w279 -> [w289 _ w339]
              tunnel: w278 -> [_ w313 w338]
              tunnel: w277 -> [_ w312 w337]
              tunnel: w276 -> [_ w311 w336]
              tunnel: w275 -> [_ w310 w335]
              tunnel: w274 -> [_ w309 w334]
              frame #0 {
                n188 = Select(t=2, s=w290, f=0) -> (s? t:f=w285:i32)
                n189 = Select(t=2, s=w291, f=0) -> (s? t:f=w286:i32)
                n190 = Select(t=2, s=w289, f=0) -> (s? t:f=w284:i32)
                n191 = Select(t=2, s=w293, f=0) -> (s? t:f=w288:i32)
                n192 = Select(t=2, s=w292, f=0) -> (s? t:f=w287:i32)
                n193 = property on="LAB02-2 SELECT" class="RadioBtnsControl (strict)"("DisabledEnum"=w285) -> ()  [unwired: 2 in, 2 out]
                n194 = property on="LAB02-1 SELECT" class="RadioBtnsControl (strict)"("DisabledEnum"=w286) -> ()  [unwired: 2 in, 2 out]
                n195 = property on="LAB03-1 SELECT" class="RadioBtnsControl (strict)"("DisabledEnum"=w284) -> ()  [unwired: 2 in, 2 out]
                n196 = property on="LAB01-1 SELECT" class="RadioBtnsControl (strict)"("DisabledEnum"=w288) -> ()  [unwired: 2 in, 2 out]
                n197 = property on="LAB01-2 SELECT" class="RadioBtnsControl (strict)"("DisabledEnum"=w287) -> ()  [unwired: 2 in, 2 out]
                n198 = property on="LAB01-2 (RESULT)" class="Bool (strict)"("DisabledEnum"=w287) -> ()  [unwired: 2 in, 2 out]
                n199 = property on="LAB02-1 (RESULT)" class="Bool (strict)"("DisabledEnum"=w286) -> ()  [unwired: 2 in, 2 out]
                n200 = property on="LAB01-1 (RESULT)" class="Bool (strict)"("DisabledEnum"=w288) -> ()  [unwired: 2 in, 2 out]
                n201 = property on="LAB02-2 (RESULT)" class="Bool (strict)"("DisabledEnum"=w285) -> ()  [unwired: 2 in, 2 out]
                n202 = property on="LAB03-1 (RESULT)" class="Bool (strict)"("DisabledEnum"=w284) -> ()  [unwired: 2 in, 2 out]
              }
              frame #1 {
                n203 = Select(t=2, s=w309, f=0) -> (s? t:f=w304:i32)
                n204 = Select(t=2, s=w310, f=0) -> (s? t:f=w305:i32)
                n205 = Select(t=2, s=w313, f=0) -> (s? t:f=w308:i32)
                n206 = Select(t=2, s=w312, f=0) -> (s? t:f=w307:i32)
                n207 = Select(t=2, s=w311, f=0) -> (s? t:f=w306:i32)
                n208 = property on="LAB05-2 SELECT" class="RadioBtnsControl (strict)"("DisabledEnum"=w304) -> ()  [unwired: 2 in, 2 out]
                n209 = property on="LAB05-1 SELECT" class="RadioBtnsControl (strict)"("DisabledEnum"=w305) -> ()  [unwired: 2 in, 2 out]
                n210 = property on="LAB03-2 SELECT" class="RadioBtnsControl (strict)"("DisabledEnum"=w308) -> ()  [unwired: 2 in, 2 out]
                n211 = property on="LAB04-1 SELECT" class="RadioBtnsControl (strict)"("DisabledEnum"=w307) -> ()  [unwired: 2 in, 2 out]
                n212 = property on="LAB04-2 SELECT" class="RadioBtnsControl (strict)"("DisabledEnum"=w306) -> ()  [unwired: 2 in, 2 out]
                n213 = property on="LAB05-2 (RESULT)" class="Bool (strict)"("DisabledEnum"=w304) -> ()  [unwired: 2 in, 2 out]
                n214 = property on="LAB05-1 (RESULT)" class="Bool (strict)"("DisabledEnum"=w305) -> ()  [unwired: 2 in, 2 out]
                n215 = property on="LAB04-2 (RESULT)" class="Bool (strict)"("DisabledEnum"=w306) -> ()  [unwired: 2 in, 2 out]
                n216 = property on="LAB04-1 (RESULT)" class="Bool (strict)"("DisabledEnum"=w307) -> ()  [unwired: 2 in, 2 out]
                n217 = property on="LAB03-2 (RESULT)" class="Bool (strict)"("DisabledEnum"=w308) -> ()  [unwired: 2 in, 2 out]
              }
              frame #2 {
                # "disable calibrate if any test running"
                n218 = Or(x=w335, y=w334) -> (x .or. y?=w328:bool)
                n219 = Or(x=w337, y=w336) -> (x .or. y?=w330:bool)
                n220 = Or(x=w341, y=w340) -> (x .or. y?=w332:bool)
                n221 = Or(x=w339, y=w338) -> (x .or. y?=w331:bool)
                n222 = Or(x=w343, y=w342) -> (x .or. y?=w333:bool)
                n223 = Or(x=w331, y=w330) -> (x .or. y?=w329:bool)
                n224 = Or(x=w333, y=w332) -> (x .or. y?=w327:bool)
                n225 = Or(x=w329, y=w328) -> (x .or. y?=w326:bool)
                n226 = Or(x=w327, y=w326) -> (x .or. y?=w325:bool)
                n227 = case shown="False" w325 {
                  tunnel: [0 2] -> w324
                  frame False {
                  }
                  frame True {
                  }
                }
                n228 = property on="CALIBRATE" class="Bool (strict)"("DisabledEnum"=w324) -> ()  [unwired: 2 in, 2 out]
              }
            }
          }
          frame #6 {
            # "check for RUN switch change, start test if true and stop test if false"
            n229 = Get Date/Time In Seconds() -> (seconds since 1Jan1904=w350:timestamp)
            n230 = Format Date/Time String(time format string (%c)="%Y%m%d", seconds (now)=w350) -> (date/time string=w351:string)  [unwired: 1 in]
            n231 = Format Date/Time String(time format string (%c)="%H%M", seconds (now)=w350) -> (date/time string=w348:string)  [unwired: 1 in]
            n232 = event shown="[1] \"LAB01-1RUN\": Value Change" {
              selector: _ -> [_ _]
              dyn-events: _ -> [_ _]
              timeout: 10 -> [_ _]
              tunnel: "c:\\crabtree\\Test Data\\" -> [_ w359]
              tunnel: w351 -> [_ w358]
              tunnel: w348 -> [_ w356]
              tunnel: w347 -> [_ w357]
              tunnel: w346 -> [_ w355]
              event Timeout {
                n233 = event-data() -> ()  [unwired: 1 in, 3 out]
              }
              event "LAB01-1RUN": Value Change {
                n234 = event-data() -> ()  [unwired: 1 in, 6 out]
                n235 = case shown="True" w355 {
                  tunnel: w359 -> [_ w382]
                  tunnel: w358 -> [_ w381]
                  tunnel: w357 -> [w360 w380]
                  tunnel: w356 -> [_ w379]
                  tunnel: w355 -> [_ w378]
                  frame False {
                    # "stop test"
                    n236 = stacked-sequence {
                      tunnel: w360 -> [w366 _]
                      frame #0 {
                        n237 = local read "LAB01 (DISP 1)"() -> (w365:T5)
                        n238 = Unbundle(w365) -> ("1 (CYCLE)"=w363:dbl, "1 (T-RISE min)"=w364:dbl)  [unwired: 4 out]
                        n239 = case shown="\"CYCLE TEST\"" w366 {
                          tunnel: w364 -> [_ _ w373]
                          tunnel: w363 -> [w371 w372 _]
                          tunnel: [w371 w372 w373] -> w362
                          frame "TEST SET UP", Default {
                          }
                          frame "CYCLE TEST" {
                          }
                          frame "T-RISE TEST" {
                          }
                        }
                        n240 = local read "LAB01-1 (TDMS)"() -> (w370:refnum<k34>)
                        n241 = Build Array("STOPPED") -> (w367:string[])
                        n242 = Build Array(w362) -> (w361:dbl[])
                        n243 = TDMS Write(0:w370, 5:"TEST RESULT", 7:w367, 9:w361) -> ()  [unwired: 2 in, 4 out]
                      }
                      frame #1 {
                        n244 = local read "LAB01 (DISP 1)"() -> (w377:T5)
                        n245 = Bundle(cluster=w377, "1 (STATUS)"="STOP") -> (w375:T5)  [unwired: 5 in]
                        n246 = local write "LAB01-1 (RESULT)"(FALSE) -> ()
                        n247 = local write "LAB01 (DISP 1)"(w375) -> ()
                      }
                    }
                  }
                  frame True {
                    # "start new test and create test file"
                    n248 = stacked-sequence {
                      seq-local: [w388 _ _ _ _] -> [_ w401 _ _ _]
                      tunnel: w382 -> [w397 _ _ _ _]
                      tunnel: w381 -> [w395 _ _ _ _]
                      tunnel: w380 -> [w394 _ _ _ _]
                      tunnel: w379 -> [w385 _ _ _ _]
                      tunnel: w378 -> [_ w402 _ _ _]
                      frame #0 {
                        n249 = local read "LAB01 (SETTINGS 1)"() -> (w387:T4)
                        n250 = case shown="\"TEST SET UP\", Default" w394 {
                          tunnel: ["TEST SET UP-" "CYCLE TEST-" "T-RISE TEST-"] -> w390
                          frame "TEST SET UP", Default {
                          }
                          frame "CYCLE TEST" {
                          }
                          frame "T-RISE TEST" {
                          }
                        }
                        n251 = Unbundle(w387) -> ("1 Description"=w386:string)  [unwired: 9 out]
                        n252 = Concatenate Strings(w397, "LAB01-1\\", w395, "\\") -> (w391:string)
                        n253 = String To Path(string=w391) -> (path=w393:path)
                        n254 = Concatenate Strings(w391, w390, w386, "-", w385, ".tdms") -> (w388:string)
                        n255 = Create Folder(path (use dialog)=w393) -> (error out=w392:errorcluster)  [unwired: 2 in, 2 out]
                        n256 = call <vilib>:"Clear Errors.vi"("error in (no error)"=w392) -> ()  [unwired: 6 in, 1 out]
                      }
                      frame #1 {
                        n257 = case shown="True" w402 {
                          tunnel: w401 -> [_ w403]
                          frame False {
                          }
                          frame True {
                            n258 = String To Path(string=w403) -> (path=w404:path)
                            n259 = TDMS Open(5:FALSE, 6:FALSE, 10:T14."create or replace" ("operation (0:open)"), 11:w404) -> (0:w406:errorcluster, 3:→"LAB01-1 (TDMS)":refnum<k34>)  [unwired: 3 in]
                            n260 = local write "data file error"(w406) -> ()
                          }
                        }
                      }
                      frame #2 {
                        n261 = local read "LAB01 (SETTINGS 1)"() -> (w415:T4)
                        n262 = local read "LAB01-1 (TDMS)"() -> (w426:refnum<k34>)
                        n263 = Build Array("Testers Name", "Description", "Set Test Cycles", "T-Rise minutes", "T-Rise Deg C") -> (w416:string[])
                        n264 = Unbundle(w415) -> ("1 Name"=w414:string, "1 Description"=w413:string, "1 (CYCLES)"=w412:dbl, "1 (T-RISE mins)"=w411:dbl, "1 (T-RISE deg C)"=w410:dbl)  [unwired: 5 out]
                        n265 = Number To Decimal String(number=w412) -> (decimal integer string=w425:string)  [unwired: 1 in]
                        n266 = Number To Decimal String(number=w411) -> (decimal integer string=w424:string)  [unwired: 1 in]
                        n267 = Number To Decimal String(number=w410) -> (decimal integer string=w423:string)  [unwired: 1 in]
                        n268 = Build Array(w414, w413, w425, w424, w423) -> (w422:string[])
                        n269 = TDMS Set Properties(5:w422, 7:w416, 11:w426) -> ()  [unwired: 3 in, 4 out]
                      }
                      frame #3 {
                        w428 = 0.0
                        n270 = local read "LAB01 (DISP 1)"() -> (w430:T5)
                        n271 = Bundle(cluster=w430, "1 (CYCLE)"=w428, "1 (T-RISE min)"=w428, "1 (STATUS)"="RUN") -> (w429:T5)  [unwired: 3 in]
                        n272 = local write "LAB01 (DISP 1)"(w429) -> ()
                      }
                      frame #4 {
                        n273 = local read "LAB01-1 (SIG)"() -> (w433:T2)
                        n274 = local read "LAB01 (TEMP START)"() -> (w435:T6)
                        n275 = Unbundle(w433) -> ("Tmp Live"=w432:dbl, "Tmp Neut"=w431:dbl)  [unwired: 3 out]
                        n276 = Bundle(cluster=w435, "1 (TL)"=w432, "1 (TN)"=w431) -> (w434:T6)  [unwired: 2 in]
                        n277 = local write "LAB01 (TEMP START)"(w434) -> ()
                      }
                    }
                  }
                }
              }
            }
          }
          frame #7 {
            # "end test & close test files"
            n278 = stacked-sequence {
              frame #0 {
                n279 = local read "LAB01 (DISP 1)"() -> (w437:T5)
                n280 = Unbundle(w437) -> ("1 (STATUS)"=w436:string)  [unwired: 5 out]
                n281 = Equal?(x=w436, y="STOP") -> (x = y?=w438:bool)
                n282 = case shown="True" w438 {
                  frame False {
                  }
                  frame True {
                    n283 = stacked-sequence {
                      frame #0 {
                        n284 = local read "LAB01 (DISP 1)"() -> (w442:T5)
                        n285 = Bundle(cluster=w442, "1 (STATUS)"="END") -> (w440:T5)  [unwired: 5 in]
                        n286 = local write "LAB01 (DISP 1)"(w440) -> ()
                      }
                      frame #1 {
                        n287 = local read "LAB01-1 (TDMS)"() -> (w445:refnum<k34>)
                        n288 = TDMS Close(11:w445) -> (0:w444:errorcluster)  [unwired: 1 in, 1 out]
                        n289 = local write "LAB01-1RUN"(FALSE) -> ()
                        n290 = local write "data file error"(w444) -> ()
                      }
                    }
                  }
                }
              }
            }
          }
          frame #8 {
            # "drive jigs"
            n291 = stacked-sequence {
              frame #0 {
                # "jig on"
                n292 = local read "jig cycle"() -> (w446:dbl)
                n293 = Equal?(x=w446, y=0) -> (x = y?=w448:bool)
                n294 = case shown="True" w448 {
                  frame False {
                  }
                  frame True {
                    n295 = local read "LAB01-1RUN"() -> (w449:bool)
                    n296 = local read "LAB01-2 RUN"() -> (w450:bool)
                    n297 = local read "LAB03-1 RUN"() -> (w456:bool)
                    n298 = local read "LAB03-2 RUN"() -> (w455:bool)
                    n299 = local read "LAB02-1 RUN"() -> (w458:bool)
                    n300 = local read "LAB02-2 RUN"() -> (w457:bool)
                    n301 = local read "LAB04-1 RUN"() -> (w454:bool)
                    n302 = local read "LAB04-2 RUN"() -> (w453:bool)
                    n303 = local read "LAB05-1 RUN"() -> (w452:bool)
                    n304 = local read "LAB05-2 RUN"() -> (w451:bool)
                    n305 = local write "LAB05-1 (JIG)"(w452) -> ()
                    n306 = local write "LAB05-2 (JIG)"(w451) -> ()
                    n307 = local write "LAB04-2 (JIG)"(w453) -> ()
                    n308 = local write "LAB02-1 (JIG)"(w458) -> ()
                    n309 = local write "LAB03-1 (JIG)"(w456) -> ()
                    n310 = local write "LAB04-1 (JIG)"(w454) -> ()
                    n311 = local write "LAB03-2 (JIG)"(w455) -> ()
                    n312 = local write "LAB02-2 (JIG)"(w457) -> ()
                    n313 = local write "LAB01-1 (JIG)"(w449) -> ()
                    n314 = local write "LAB01-2 (JIG)"(w450) -> ()
                  }
                }
              }
              frame #1 {
                # "jig off"
                n315 = local read "jig cycle"() -> (w461:dbl)
                n316 = local read "on loops"() -> (w460:dbl)
                n317 = Equal?(x=w461, y=w460) -> (x = y?=w459:bool)
                n318 = case shown="True" w459 {
                  frame False {
                  }
                  frame True {
                    w512 = FALSE
                    w513 = TRUE
                    w511 = 2
                    n319 = local read "LAB05-2 SELECT"() -> (w502:T3)
                    n320 = local read "LAB04-2 SELECT"() -> (w504:T3)
                    n321 = local read "LAB04-1 SELECT"() -> (w505:T3)
                    n322 = local read "LAB05-1 SELECT"() -> (w503:T3)
                    n323 = local read "LAB03-2 SELECT"() -> (w506:T3)
                    n324 = local read "LAB02-1 SELECT"() -> (w509:T3)
                    n325 = local read "LAB03-1 SELECT"() -> (w507:T3)
                    n326 = local read "LAB02-2 SELECT"() -> (w508:T3)
                    n327 = local read "LAB01-2 SELECT"() -> (w510:T3)
                    n328 = local read "LAB05-1 RUN"() -> (w472:bool)
                    n329 = local read "LAB05-2 RUN"() -> (w471:bool)
                    n330 = local read "LAB04-2 RUN"() -> (w473:bool)
                    n331 = local read "LAB04-1 RUN"() -> (w474:bool)
                    n332 = local read "LAB01-2 RUN"() -> (w479:bool)
                    n333 = local read "LAB03-2 RUN"() -> (w475:bool)
                    n334 = local read "LAB01-1RUN"() -> (w490:bool)
                    n335 = local read "LAB01-1 SELECT"() -> (w514:T3)
                    n336 = local read "LAB03-1 RUN"() -> (w476:bool)
                    n337 = local read "LAB02-1 RUN"() -> (w478:bool)
                    n338 = local read "LAB02-2 RUN"() -> (w477:bool)
                    n339 = Equal?(x=w511, y=w507) -> (x = y?=w485:bool)
                    n340 = Equal?(x=w511, y=w506) -> (x = y?=w484:bool)
                    n341 = Equal?(x=w511, y=w505) -> (x = y?=w483:bool)
                    n342 = Equal?(x=w511, y=w504) -> (x = y?=w482:bool)
                    n343 = Equal?(x=w511, y=w503) -> (x = y?=w481:bool)
                    n344 = Equal?(x=w511, y=w502) -> (x = y?=w480:bool)
                    n345 = Equal?(x=w511, y=w514) -> (x = y?=w491:bool)
                    n346 = Equal?(x=w511, y=w509) -> (x = y?=w487:bool)
                    n347 = Equal?(x=w511, y=w508) -> (x = y?=w486:bool)
                    n348 = Equal?(x=w511, y=w510) -> (x = y?=w488:bool)
                    n349 = And(x=w482, y=w473) -> (x .and. y?=w464:bool)
                    n350 = And(x=w485, y=w476) -> (x .and. y?=w467:bool)
                    n351 = And(x=w483, y=w474) -> (x .and. y?=w465:bool)
                    n352 = And(x=w480, y=w471) -> (x .and. y?=w462:bool)
                    n353 = And(x=w486, y=w477) -> (x .and. y?=w468:bool)
                    n354 = And(x=w484, y=w475) -> (x .and. y?=w466:bool)
                    n355 = And(x=w481, y=w472) -> (x .and. y?=w463:bool)
                    n356 = And(x=w488, y=w479) -> (x .and. y?=w470:bool)
                    n357 = And(x=w491, y=w490) -> (x .and. y?=w489:bool)
                    n358 = And(x=w487, y=w478) -> (x .and. y?=w469:bool)
                    n359 = Select(t=w513, s=w489, f=w512) -> (s? t:f=w492:bool)
                    n360 = Select(t=w513, s=w470, f=w512) -> (s? t:f=w493:bool)
                    n361 = Select(t=w513, s=w469, f=w512) -> (s? t:f=w494:bool)
                    n362 = Select(t=w513, s=w468, f=w512) -> (s? t:f=w495:bool)
                    n363 = Select(t=w513, s=w467, f=w512) -> (s? t:f=w496:bool)
                    n364 = Select(t=w513, s=w466, f=w512) -> (s? t:f=w497:bool)
                    n365 = Select(t=w513, s=w465, f=w512) -> (s? t:f=w498:bool)
                    n366 = Select(t=w513, s=w464, f=w512) -> (s? t:f=w499:bool)
                    n367 = Select(t=w513, s=w463, f=w512) -> (s? t:f=w500:bool)
                    n368 = Select(t=w513, s=w462, f=w512) -> (s? t:f=w501:bool)
                    n369 = local write "LAB03-2 (JIG)"(w497) -> ()
                    n370 = local write "LAB02-1 (JIG)"(w494) -> ()
                    n371 = local write "LAB02-2 (JIG)"(w495) -> ()
                    n372 = local write "LAB01-2 (JIG)"(w493) -> ()
                    n373 = local write "LAB03-1 (JIG)"(w496) -> ()
                    n374 = local write "LAB01-1 (JIG)"(w492) -> ()
                    n375 = local write "LAB05-2 (JIG)"(w501) -> ()
                    n376 = local write "LAB04-1 (JIG)"(w498) -> ()
                    n377 = local write "LAB05-1 (JIG)"(w500) -> ()
                    n378 = local write "LAB04-2 (JIG)"(w499) -> ()
                  }
                }
              }
            }
          }
          frame #9 {
            # "drive digital output"
            n379 = local read "LAB05-2 (O/I)"() -> (w520:bool)
            n380 = local read "LAB05-2 (JIG)"() -> (w519:bool)
            n381 = local read "LAB05-1 (O/I)"() -> (w522:bool)
            n382 = local read "LAB05-1 (JIG)"() -> (w521:bool)
            n383 = local read "LAB04-2 (O/I)"() -> (w524:bool)
            n384 = local read "LAB04-2 (JIG)"() -> (w523:bool)
            n385 = local read "LAB03-1 (O/I)"() -> (w529:bool)
            n386 = local read "LAB04-1 (O/I)"() -> (w525:bool)
            n387 = local read "LAB04-1 (JIG)"() -> (w518:bool)
            n388 = local read "LAB02-1 (O/I)"() -> (w533:bool)
            n389 = local read "LAB02-2 (O/I)"() -> (w531:bool)
            n390 = local read "LAB03-2 (O/I)"() -> (w527:bool)
            n391 = local read "LAB03-2 (JIG)"() -> (w526:bool)
            n392 = local read "LAB02-1 (JIG)"() -> (w532:bool)
            n393 = local read "LAB02-2 (JIG)"() -> (w530:bool)
            n394 = local read "LAB03-1 (JIG)"() -> (w528:bool)
            n395 = local read "LAB01-2 (O/I)"() -> (w535:bool)
            n396 = local read "LAB01-2 (JIG)"() -> (w534:bool)
            n397 = local read "LAB01-1 (O/I)"() -> (w537:bool)
            n398 = local read "LAB01-1 (JIG)"() -> (w536:bool)
            n399 = Build Array(w524, w523, w522, w521, w520, w519) -> (w515:bool[])
            n400 = Build Array(w530, w529, w528, w527, w526, w525, w518) -> (w516:bool[])
            n401 = Build Array(w537, w536, w535, w534, w533, w532, w531) -> (w517:bool[])
            n402 = call "sub vi - Drive Relays All v6.vi"("Array #2"=w515, "Array #1"=w516, "Array #0"=w517) -> ()  [unwired: 8 in, 1 out]
          }
          frame #10 {
            # "get temperature values"
            n403 = stacked-sequence {
              frame #0 {
                n404 = local read "jig cycle"() -> (w538:dbl)
                n405 = local read "on loops"() -> (w541:dbl)
                n406 = local read "jig cycle"() -> (w543:dbl)
                n407 = Add(x=w541, y=1) -> (x+y=w542:dbl)
                n408 = Equal?(x=w543, y=0) -> (x = y?=w544:bool)
                n409 = Equal?(x=w538, y=w542) -> (x = y?=w539:bool)
                n410 = case shown="True" w544 {
                  frame False {
                  }
                  frame True {
                    w556 = FALSE
                    w557 = TRUE
                    n411 = local write "TEMP update"(TRUE) -> ()
                    n412 = call "sub vi - GET ALL TEMP v3.vi"("LA01-EN"=w557, "LA02-EN"=w557, "LA03-EN"=w557, "LA04-EN"=w556, "LA05-EN"=w556, "Gen Cal Value"=1.0) -> ("LA01 TEMP"=w555:T15, "LA02 TEMP"=w553:T15, "LA03 TEMP"=w552:T15)  [unwired: 4 in, 3 out]
                    n413 = local write "LAB03 TEMP"(w552) -> ()
                    n414 = local write "LAB02 TEMP"(w553) -> ()
                    n415 = local write "LAB01 TEMP"(w555) -> ()
                  }
                }
                n416 = case shown="True" w539 {
                  frame False {
                  }
                  frame True {
                    w549 = TRUE
                    w550 = FALSE
                    n417 = local write "TEMP update"(TRUE) -> ()
                    n418 = call "sub vi - GET ALL TEMP v3.vi"("LA01-EN"=w550, "LA02-EN"=w550, "LA03-EN"=w550, "LA04-EN"=w549, "LA05-EN"=w549, "Gen Cal Value"=1.0) -> ("LA04 TEMP"=w547:T15, "LA05 TEMP"=w546:T15)  [unwired: 4 in, 4 out]
                    n419 = local write "LAB04 TEMP"(w547) -> ()
                    n420 = local write "LAB05 TEMP"(w546) -> ()
                  }
                }
              }
              frame #1 {
                n421 = local read "LAB01 (CAL)"() -> (w575:T7)
                n422 = local read "LAB01 TEMP"() -> (w576:T10)
                n423 = Unbundle By Name(w576) -> ("T1 Live"=w566:dbl, "T1 Neut"=w565:dbl, "T2 Live"=w564:dbl, "T2 Neut"=w563:dbl)  [unwired: 2 out]
                n424 = Unbundle By Name(w575) -> ("1 (TL) cal"=w562:dbl, "1 (TN) cal"=w561:dbl, "2 (TL) cal"=w560:dbl, "2 (TN) cal"=w559:dbl)  [unwired: 6 out]
                n425 = Multiply(x=w566, y=w562) -> (x*y=w572:dbl)
                n426 = Multiply(x=w565, y=w561) -> (x*y=w571:dbl)
                n427 = Multiply(x=w564, y=w560) -> (x*y=w568:dbl)
                n428 = Multiply(x=w563, y=w559) -> (x*y=w567:dbl)
                n429 = local read "LAB01-2 (SIG)"() -> (w570:T2)
                n430 = local read "LAB01-1 (SIG)"() -> (w574:T2)
                n431 = Bundle By Name(cluster=w574, "Tmp Live"=w572, "Tmp Neut"=w571) -> (w573:T2)
                n432 = Bundle By Name(cluster=w570, "Tmp Live"=w568, "Tmp Neut"=w567) -> (w569:T2)
                n433 = local write "LAB01-1 (SIG)"(w573) -> ()
                n434 = local write "LAB01-2 (SIG)"(w569) -> ()
              }
              frame #2 {
                n435 = local read "LAB02 (CAL)"() -> (w593:T8)
                n436 = local read "LAB02 TEMP"() -> (w594:T10)
                n437 = Unbundle By Name(w594) -> ("T1 Live"=w584:dbl, "T1 Neut"=w583:dbl, "T2 Live"=w582:dbl, "T2 Neut"=w581:dbl)  [unwired: 2 out]
                n438 = Unbundle By Name(w593) -> ("1 (TL) cal"=w580:dbl, "1 (TN) cal"=w579:dbl, "2 (TL) cal"=w578:dbl, "2 (TN) cal"=w577:dbl)  [unwired: 6 out]
                n439 = Multiply(x=w584, y=w580) -> (x*y=w590:dbl)
                n440 = Multiply(x=w583, y=w579) -> (x*y=w589:dbl)
                n441 = Multiply(x=w582, y=w578) -> (x*y=w586:dbl)
                n442 = Multiply(x=w581, y=w577) -> (x*y=w585:dbl)
                n443 = local read "LAB02-2 (SIG)"() -> (w588:T2)
                n444 = local read "LAB02-1 (SIG)"() -> (w592:T2)
                n445 = Bundle By Name(cluster=w592, "Tmp Live"=w590, "Tmp Neut"=w589) -> (w591:T2)
                n446 = Bundle By Name(cluster=w588, "Tmp Live"=w586, "Tmp Neut"=w585) -> (w587:T2)
                n447 = local write "LAB02-1 (SIG)"(w591) -> ()
                n448 = local write "LAB02-2 (SIG)"(w587) -> ()
              }
              frame #3 {
                n449 = local read "LAB03 (CAL)"() -> (w611:T7)
                n450 = local read "LAB03 TEMP"() -> (w612:T10)
                n451 = Unbundle By Name(w612) -> ("T1 Live"=w602:dbl, "T1 Neut"=w601:dbl, "T2 Live"=w600:dbl, "T2 Neut"=w599:dbl)  [unwired: 2 out]
                n452 = Unbundle By Name(w611) -> ("1 (TL) cal"=w598:dbl, "1 (TN) cal"=w597:dbl, "2 (TL) cal"=w596:dbl, "2 (TN) cal"=w595:dbl)  [unwired: 6 out]
                n453 = Multiply(x=w602, y=w598) -> (x*y=w608:dbl)
                n454 = Multiply(x=w601, y=w597) -> (x*y=w607:dbl)
                n455 = Multiply(x=w600, y=w596) -> (x*y=w604:dbl)
                n456 = Multiply(x=w599, y=w595) -> (x*y=w603:dbl)
                n457 = local read "LAB03-2 (SIG)"() -> (w606:T2)
                n458 = local read "LAB03-1 (SIG)"() -> (w610:T2)
                n459 = Bundle By Name(cluster=w610, "Tmp Live"=w608, "Tmp Neut"=w607) -> (w609:T2)
                n460 = Bundle By Name(cluster=w606, "Tmp Live"=w604, "Tmp Neut"=w603) -> (w605:T2)
                n461 = local write "LAB03-1 (SIG)"(w609) -> ()
                n462 = local write "LAB03-2 (SIG)"(w605) -> ()
              }
              frame #4 {
                n463 = local read "LAB04 (CAL)"() -> (w629:T7)
                n464 = local read "LAB04 TEMP"() -> (w630:T10)
                n465 = Unbundle By Name(w630) -> ("T1 Live"=w620:dbl, "T1 Neut"=w619:dbl, "T2 Live"=w618:dbl, "T2 Neut"=w617:dbl)  [unwired: 2 out]
                n466 = Unbundle By Name(w629) -> ("1 (TL) cal"=w616:dbl, "1 (TN) cal"=w615:dbl, "2 (TL) cal"=w614:dbl, "2 (TN) cal"=w613:dbl)  [unwired: 6 out]
                n467 = Multiply(x=w620, y=w616) -> (x*y=w626:dbl)
                n468 = Multiply(x=w619, y=w615) -> (x*y=w625:dbl)
                n469 = Multiply(x=w618, y=w614) -> (x*y=w622:dbl)
                n470 = Multiply(x=w617, y=w613) -> (x*y=w621:dbl)
                n471 = local read "LAB04-2 (SIG)"() -> (w624:T2)
                n472 = local read "LAB04-1 (SIG)"() -> (w628:T2)
                n473 = Bundle By Name(cluster=w628, "Tmp Live"=w626, "Tmp Neut"=w625) -> (w627:T2)
                n474 = Bundle By Name(cluster=w624, "Tmp Live"=w622, "Tmp Neut"=w621) -> (w623:T2)
                n475 = local write "LAB04-1 (SIG)"(w627) -> ()
                n476 = local write "LAB04-2 (SIG)"(w623) -> ()
              }
              frame #5 {
                n477 = local read "LAB05 (CAL)"() -> (w647:T7)
                n478 = local read "LAB05 TEMP"() -> (w648:T10)
                n479 = Unbundle By Name(w648) -> ("T1 Live"=w638:dbl, "T1 Neut"=w637:dbl, "T2 Live"=w636:dbl, "T2 Neut"=w635:dbl)  [unwired: 2 out]
                n480 = Unbundle By Name(w647) -> ("1 (TL) cal"=w634:dbl, "1 (TN) cal"=w633:dbl, "2 (TL) cal"=w632:dbl, "2 (TN) cal"=w631:dbl)  [unwired: 6 out]
                n481 = Multiply(x=w638, y=w634) -> (x*y=w644:dbl)
                n482 = Multiply(x=w637, y=w633) -> (x*y=w643:dbl)
                n483 = Multiply(x=w636, y=w632) -> (x*y=w640:dbl)
                n484 = Multiply(x=w635, y=w631) -> (x*y=w639:dbl)
                n485 = local read "LAB05-2 (SIG)"() -> (w642:T2)
                n486 = local read "LAB05-1 (SIG)"() -> (w646:T2)
                n487 = Bundle By Name(cluster=w646, "Tmp Live"=w644, "Tmp Neut"=w643) -> (w645:T2)
                n488 = Bundle By Name(cluster=w642, "Tmp Live"=w640, "Tmp Neut"=w639) -> (w641:T2)
                n489 = local write "LAB05-1 (SIG)"(w645) -> ()
                n490 = local write "LAB05-2 (SIG)"(w641) -> ()
              }
            }
          }
          frame #11 {
            # "get analog values"
            n491 = local read "on loops"() -> (w655:dbl)
            n492 = local read "jig cycle"() -> (w652:dbl)
            n493 = Add(x=w655, y=2) -> (x+y=w653:dbl)
            n494 = Equal?(x=w652, y=1) -> (x = y?=w650:bool)
            n495 = Equal?(x=w652, y=w653) -> (x = y?=w651:bool)
            n496 = Or(x=w650, y=w651) -> (x .or. y?=w649:bool)
            n497 = case shown="True" w649 {
              frame False {
              }
              frame True {
                n498 = call "sub vi - Read Analog All v7.vi"() -> ("Analog loop time"=w663:dbl, "array GRAPH"=w662:dynamicdata[], "LAB01"=w661:T16, "LAB02"=w660:T17, "LAB03"=w659:T18, "LAB04"=w658:T19, "array ERROR"=w664:errorcluster[], "LAB05"=w657:T20)  [unwired: 8 in]
                n499 = stacked-sequence {
                  tunnel: w664 -> [w667 _ _ _ _ _]
                  tunnel: w663 -> [w666 _ _ _ _ _]
                  tunnel: w662 -> [w665 _ _ _ _ _]
                  tunnel: w661 -> [_ w712 _ _ _ _]
                  tunnel: w660 -> [_ _ w713 _ _ _]
                  tunnel: w659 -> [_ _ _ w737 _ _]
                  tunnel: w658 -> [_ _ _ _ w761 _]
                  tunnel: w657 -> [_ _ _ _ _ w785]
                  frame #0 {
                    n500 = local write "AI update"(TRUE) -> ()
                    n501 = Index Array(array=w665, index=6) -> (element=→"LAB04-1 (GRAPH)":dynamicdata)
                    n502 = Index Array(array=w665, index=7) -> (element=→"LAB04-2 (GRAPH)":dynamicdata)
                    n503 = Index Array(array=w665, index=9) -> (element=→"LAB05-2 (GRAPH)":dynamicdata)
                    n504 = Index Array(array=w665, index=8) -> (element=→"LAB05-1 (GRAPH)":dynamicdata)
                    n505 = Index Array(array=w665, index=5) -> (element=→"LAB03-2 (GRAPH)":dynamicdata)
                    n506 = Index Array(array=w665, index=0) -> (element=→"LAB01-1 (GRAPH)":dynamicdata)
                    n507 = Index Array(array=w665, index=1) -> (element=→"LAB01-2 (GRAPH)":dynamicdata)
                    n508 = Index Array(array=w665, index=2) -> (element=→"LAB02-1 (GRAPH)":dynamicdata)
                    n509 = Index Array(array=w665, index=3) -> (element=→"LAB02-2 (GRAPH)":dynamicdata)
                    n510 = Index Array(array=w665, index=4) -> (element=→"LAB03-1 (GRAPH)":dynamicdata)
                    "AI loop time" <- w666
                    "Analog Error Array" <- w667
                  }
                  frame #1 {
                    n511 = local read "LAB01 (CAL)"() -> (w711:T7)
                    n512 = Unbundle By Name(w712) -> ("LAB01-1 (A)"=w710:dbl, "LAB01-1 (V)"=w709:dbl, "LAB01-1 (PF)"=w708:dbl, "LAB01-2 (A)"=w707:dbl, "LAB01-2 (V)"=w706:dbl, "LAB01-2 (PF)"=w705:dbl)
                    n513 = Unbundle By Name(w711) -> ("1  (A) cal"=w704:dbl, "1 (V) cal"=w703:dbl, "1 (PF) cal"=w702:dbl, "2 (A) cal"=w701:dbl, "2 (V) cal"=w700:dbl, "2 (PF) cal"=w699:dbl)  [unwired: 4 out]
                    n514 = Multiply(x=w710, y=w704) -> (x*y=w697:dbl)
                    n515 = Multiply(x=w709, y=w703) -> (x*y=w696:dbl)
                    n516 = Multiply(x=w708, y=w702) -> (x*y=w695:dbl)
                    n517 = Multiply(x=w707, y=w701) -> (x*y=w691:dbl)
                    n518 = local read "LAB01-1 (SIG)"() -> (w698:T2)
                    n519 = Multiply(x=w706, y=w700) -> (x*y=w690:dbl)
                    n520 = Multiply(x=w705, y=w699) -> (x*y=w689:dbl)
                    n521 = local read "LAB01-2 (SIG)"() -> (w693:T2)
                    n522 = Bundle By Name(cluster=w698, "AMPS"=w697, "VOLTS"=w696, "PF"=w695) -> (w694:T2)
                    n523 = Bundle By Name(cluster=w693, "AMPS"=w691, "VOLTS"=w690, "PF"=w689) -> (w692:T2)
                    n524 = local write "LAB01-2 (SIG)"(w692) -> ()
                    n525 = local write "LAB01-1 (SIG)"(w694) -> ()
                  }
                  frame #2 {
                    n526 = local read "LAB02 (CAL)"() -> (w736:T8)
                    n527 = Unbundle By Name(w713) -> ("LAB02-1 (A)"=w735:dbl, "LAB02-1 (V)"=w734:dbl, "LAB02-1 (PF)"=w733:dbl, "LAB02-2 (A)"=w732:dbl, "LAB02-2 (V)"=w731:dbl, "LAB02-2 (PF)"=w730:dbl)
                    n528 = Unbundle By Name(w736) -> ("1 (A) cal"=w729:dbl, "1 (V) cal"=w728:dbl, "1 (PF) cal"=w727:dbl, "2 (A) cal"=w726:dbl, "2 (V) cal"=w725:dbl, "2 (PF) cal"=w724:dbl)  [unwired: 4 out]
                    n529 = Multiply(x=w735, y=w729) -> (x*y=w722:dbl)
                    n530 = Multiply(x=w734, y=w728) -> (x*y=w721:dbl)
                    n531 = Multiply(x=w733, y=w727) -> (x*y=w720:dbl)
                    n532 = Multiply(x=w732, y=w726) -> (x*y=w716:dbl)
                    n533 = local read "LAB02-1 (SIG)"() -> (w723:T2)
                    n534 = Multiply(x=w731, y=w725) -> (x*y=w715:dbl)
                    n535 = Multiply(x=w730, y=w724) -> (x*y=w714:dbl)
                    n536 = local read "LAB02-2 (SIG)"() -> (w718:T2)
                    n537 = Bundle By Name(cluster=w723, "AMPS"=w722, "VOLTS"=w721, "PF"=w720) -> (w719:T2)
                    n538 = Bundle By Name(cluster=w718, "AMPS"=w716, "VOLTS"=w715, "PF"=w714) -> (w717:T2)
                    n539 = local write "LAB02-2 (SIG)"(w717) -> ()
                    n540 = local write "LAB02-1 (SIG)"(w719) -> ()
                  }
                  frame #3 {
                    n541 = local read "LAB03 (CAL)"() -> (w760:T7)
                    n542 = Unbundle By Name(w737) -> ("LAB03-1 (A)"=w759:dbl, "LAB03-1 (V)"=w758:dbl, "LAB03-1 (PF)"=w757:dbl, "LAB03-2 (A)"=w756:dbl, "LAB03-2 (V)"=w755:dbl, "LAB03-2 (PF)"=w754:dbl)
                    n543 = Unbundle By Name(w760) -> ("1  (A) cal"=w753:dbl, "1 (V) cal"=w752:dbl, "1 (PF) cal"=w751:dbl, "2 (A) cal"=w750:dbl, "2 (V) cal"=w749:dbl, "2 (PF) cal"=w748:dbl)  [unwired: 4 out]
                    n544 = Multiply(x=w759, y=w753) -> (x*y=w746:dbl)
                    n545 = Multiply(x=w758, y=w752) -> (x*y=w745:dbl)
                    n546 = Multiply(x=w757, y=w751) -> (x*y=w744:dbl)
                    n547 = Multiply(x=w756, y=w750) -> (x*y=w740:dbl)
                    n548 = local read "LAB03-1 (SIG)"() -> (w747:T2)
                    n549 = Multiply(x=w755, y=w749) -> (x*y=w739:dbl)
                    n550 = Multiply(x=w754, y=w748) -> (x*y=w738:dbl)
                    n551 = local read "LAB03-1 (SIG)"() -> (w742:T2)
                    n552 = Bundle By Name(cluster=w747, "AMPS"=w746, "VOLTS"=w745, "PF"=w744) -> (w743:T2)
                    n553 = Bundle By Name(cluster=w742, "AMPS"=w740, "VOLTS"=w739, "PF"=w738) -> (w741:T2)
                    n554 = local write "LAB03-1 (SIG)"(w741) -> ()
                    n555 = local write "LAB03-1 (SIG)"(w743) -> ()
                  }
                  frame #4 {
                    n556 = local read "LAB04 (CAL)"() -> (w784:T7)
                    n557 = Unbundle By Name(w761) -> ("LAB04-1 (A)"=w783:dbl, "LAB04-1 (V)"=w782:dbl, "LAB04-1 (PF)"=w781:dbl, "LAB04-2 (A)"=w780:dbl, "LAB04-2 (V)"=w779:dbl, "LAB04-2 (PF)"=w778:dbl)
                    n558 = Unbundle By Name(w784) -> ("1  (A) cal"=w777:dbl, "1 (V) cal"=w776:dbl, "1 (PF) cal"=w775:dbl, "2 (A) cal"=w774:dbl, "2 (V) cal"=w773:dbl, "2 (PF) cal"=w772:dbl)  [unwired: 4 out]
                    n559 = Multiply(x=w783, y=w777) -> (x*y=w770:dbl)
                    n560 = Multiply(x=w782, y=w776) -> (x*y=w769:dbl)
                    n561 = Multiply(x=w781, y=w775) -> (x*y=w768:dbl)
                    n562 = Multiply(x=w780, y=w774) -> (x*y=w764:dbl)
                    n563 = local read "LAB04-1 (SIG)"() -> (w771:T2)
                    n564 = Multiply(x=w779, y=w773) -> (x*y=w763:dbl)
                    n565 = Multiply(x=w778, y=w772) -> (x*y=w762:dbl)
                    n566 = local read "LAB04-2 (SIG)"() -> (w766:T2)
                    n567 = Bundle By Name(cluster=w771, "AMPS"=w770, "VOLTS"=w769, "PF"=w768) -> (w767:T2)
                    n568 = Bundle By Name(cluster=w766, "AMPS"=w764, "VOLTS"=w763, "PF"=w762) -> (w765:T2)
                    n569 = local write "LAB04-2 (SIG)"(w765) -> ()
                    n570 = local write "LAB04-1 (SIG)"(w767) -> ()
                  }
                  frame #5 {
                    n571 = local read "LAB05 (CAL)"() -> (w808:T7)
                    n572 = Unbundle By Name(w785) -> ("LAB05-1 (A)"=w807:dbl, "LAB05-1 (V)"=w806:dbl, "LAB05-1 (PF)"=w805:dbl, "LAB05-2 (A)"=w804:dbl, "LAB05-2 (V)"=w803:dbl, "LAB05-2 (PF)"=w802:dbl)
                    n573 = Unbundle By Name(w808) -> ("1  (A) cal"=w801:dbl, "1 (V) cal"=w800:dbl, "1 (PF) cal"=w799:dbl, "2 (A) cal"=w798:dbl, "2 (V) cal"=w797:dbl, "2 (PF) cal"=w796:dbl)  [unwired: 4 out]
                    n574 = Multiply(x=w807, y=w801) -> (x*y=w794:dbl)
                    n575 = Multiply(x=w806, y=w800) -> (x*y=w793:dbl)
                    n576 = Multiply(x=w805, y=w799) -> (x*y=w792:dbl)
                    n577 = Multiply(x=w804, y=w798) -> (x*y=w788:dbl)
                    n578 = local read "LAB05-1 (SIG)"() -> (w795:T2)
                    n579 = Multiply(x=w803, y=w797) -> (x*y=w787:dbl)
                    n580 = Multiply(x=w802, y=w796) -> (x*y=w786:dbl)
                    n581 = local read "LAB05-2 (SIG)"() -> (w790:T2)
                    n582 = Bundle By Name(cluster=w795, "AMPS"=w794, "VOLTS"=w793, "PF"=w792) -> (w791:T2)
                    n583 = Bundle By Name(cluster=w790, "AMPS"=w788, "VOLTS"=w787, "PF"=w786) -> (w789:T2)
                    n584 = local write "LAB05-2 (SIG)"(w789) -> ()
                    n585 = local write "LAB05-1 (SIG)"(w791) -> ()
                  }
                }
              }
            }
          }
          frame #12 {
            # "save test data to file"
            n586 = local read "on loops"() -> (w816:dbl)
            n587 = local read "jig cycle"() -> (w813:dbl)
            n588 = Add(x=w816, y=2) -> (x+y=w814:dbl)
            n589 = Equal?(x=w813, y=1) -> (x = y?=w811:bool)
            n590 = Equal?(x=w813, y=w814) -> (x = y?=w812:bool)
            n591 = Or(x=w811, y=w812) -> (x .or. y?=w810:bool)
            n592 = case shown="True" w810 {
              tunnel: w809 -> [_ w818]
              frame False {
              }
              frame True {
                n593 = stacked-sequence {
                  tunnel: w818 -> [w819]
                  frame #0 {
                    # "LAB01-1"
                    n594 = case shown="True" w819 {
                      frame False {
                      }
                      frame True {
                        n595 = local read "LAB01 (DISP 1)"() -> (w861:T5)
                        n596 = local read "LAB01-1 (SIG)"() -> (w862:T2)
                        n597 = local read "LAB01-1 (TDMS)"() -> (w863:refnum<k34>)
                        n598 = Build Array("TEMP Neut") -> (w827:string[])
                        n599 = Build Array("CYCLE") -> (w822:string[])
                        n600 = Build Array("TEMP Live") -> (w832:string[])
                        n601 = Build Array("PF") -> (w837:string[])
                        n602 = Build Array("AMPS") -> (w858:string[])
                        n603 = Build Array("VOLTS") -> (w849:string[])
                        n604 = Unbundle(w862) -> ("AMPS"=w857:dbl, "VOLTS"=w846:dbl, "PF"=w845:dbl, "Tmp Live"=w844:dbl, "Tmp Neut"=w847:dbl)
                        n605 = Unbundle(w861) -> ("1 (CYCLE)"=w842:dbl)  [unwired: 5 out]
                        n606 = Build Array(w846) -> (w843:dbl[])
                        n607 = Build Array(w845) -> (w836:dbl[])
                        n608 = Build Array(w844) -> (w831:dbl[])
                        n609 = Build Array(w847) -> (w826:dbl[])
                        n610 = Build Array(w857) -> (w856:dbl[])
                        n611 = Build Array(w842) -> (w821:dbl[])
                        n612 = TDMS Write(0:w863, 5:"LAB01-1 TEST VALUES", 7:w858, 9:w856) -> (4:w851:refnum<k34>, 6:w850:string, 15:w838:errorcluster)  [unwired: 2 in, 1 out]
                        n613 = TDMS Write(0:w851, 5:w850, 7:w849, 9:w843, 11:w838) -> (4:w841:refnum<k34>, 6:w840:string, 15:w839:errorcluster)  [unwired: 1 in, 1 out]
                        n614 = TDMS Write(0:w841, 5:w840, 7:w837, 9:w836, 11:w839) -> (4:w835:refnum<k34>, 6:w834:string, 15:w833:errorcluster)  [unwired: 1 in, 1 out]
                        n615 = TDMS Write(0:w835, 5:w834, 7:w832, 9:w831, 11:w833) -> (4:w830:refnum<k34>, 6:w829:string, 15:w828:errorcluster)  [unwired: 1 in, 1 out]
                        n616 = TDMS Write(0:w830, 5:w829, 7:w827, 9:w826, 11:w828) -> (4:w825:refnum<k34>, 6:w824:string, 15:w823:errorcluster)  [unwired: 1 in, 1 out]
                        n617 = TDMS Write(0:w825, 5:w824, 7:w822, 9:w821, 11:w823) -> (15:w820:errorcluster)  [unwired: 1 in, 3 out]
                        n618 = local write "data file error"(w820) -> ()
                      }
                    }
                  }
                }
              }
            }
          }
          frame #13 {
            # "check for cycle test fail conditions"
            n619 = local read "on loops"() -> (w871:dbl)
            n620 = local read "jig cycle"() -> (w868:dbl)
            n621 = local read "jig cycle"() -> (w873:dbl)
            n622 = Add(x=w871, y=2.0) -> (x+y=w869:dbl)
            n623 = Equal?(x=w873, y=1.0) -> (x = y?=w866:bool)
            n624 = Equal?(x=w868, y=w869) -> (x = y?=w864:bool)
            n625 = stacked-sequence {
              tunnel: w867 -> [w883]
              tunnel: w866 -> [w875]
              tunnel: w865 -> [w882]
              tunnel: w864 -> [w874]
              frame #0 {
                # "LAB01-1"
                n626 = case shown="\"T-RISE TEST\"" w883 {
                  tunnel: [FALSE TRUE FALSE] -> w881
                  frame "TEST SET UP", Default {
                  }
                  frame "CYCLE TEST" {
                  }
                  frame "T-RISE TEST" {
                  }
                }
                n627 = Or(x=w875, y=w874) -> (x .or. y?=w879:bool)
                n628 = local read "LAB01-1 (SIG)"() -> (w877:T2)
                n629 = And(x=w882, y=w879) -> (x .and. y?=w878:bool)
                n630 = Unbundle(w877) -> ("AMPS"=w876:dbl)  [unwired: 4 out]
                n631 = And(x=w881, y=w878) -> (x .and. y?=w880:bool)
                n632 = stacked-sequence {
                  tunnel: w880 -> [w890]
                  tunnel: w876 -> [w889]
                  tunnel: w875 -> [w888]
                  tunnel: w874 -> [w887]
                  frame #0 {
                    n633 = case shown="True" w890 {
                      tunnel: w889 -> [_ w896]
                      tunnel: w888 -> [_ w898]
                      tunnel: w887 -> [_ w897]
                      frame False {
                      }
                      frame True {
                        # "check for amps fail"
                        n634 = case shown="True" w897 {
                          tunnel: w896 -> [_ w903]
                          tunnel: [FALSE w902] -> w894
                          tunnel: ["" "AMPS HI"] -> w892
                          frame False {
                          }
                          frame True {
                            n635 = Greater?(x=w903, y=5.0) -> (0:w902:bool)
                          }
                        }
                        n636 = case shown="True" w898 {
                          tunnel: w896 -> [_ w909]
                          tunnel: [FALSE w908] -> w895
                          tunnel: ["" "AMPS LO"] -> w891
                          frame False {
                          }
                          frame True {
                            n637 = Less?(x=w909, y=5.0) -> (x < y?=w908:bool)
                          }
                        }
                        n638 = Or(x=w895, y=w894) -> (x .or. y?=w893:bool)
                        n639 = case shown="True" w893 {
                          tunnel: w892 -> [_ w912]
                          tunnel: w891 -> [_ w911]
                          frame False {
                          }
                          frame True {
                            n640 = stacked-sequence {
                              tunnel: w912 -> [w916 _]
                              tunnel: w911 -> [w915 _]
                              frame #0 {
                                n641 = local read "LAB01-1 (TDMS)"() -> (w919:refnum<k34>)
                                n642 = Build Array(w916, w915) -> (w914:string[])
                                n643 = TDMS Write(0:w919, 5:"TEST RESULT", 7:"AMPS FAIL ", 9:w914) -> (15:w918:errorcluster)  [unwired: 2 in, 3 out]
                                n644 = local write "data file error"(w918) -> ()
                              }
                              frame #1 {
                                n645 = local read "LAB01 (DISP 1)"() -> (w923:T5)
                                n646 = Bundle(cluster=w923, "1 (STATUS)"="STOP") -> (w922:T5)  [unwired: 5 in]
                                n647 = local write "LAB01-1 (RESULT)"(FALSE) -> ()
                                n648 = local write "LAB01 (DISP 1)"(w922) -> ()
                              }
                            }
                          }
                        }
                      }
                    }
                  }
                }
              }
            }
          }
          frame #14 {
            # "check for temperature rise test fail conditions"
            n649 = stacked-sequence {
              tunnel: w925 -> [w945]
              tunnel: w924 -> [w944]
              frame #0 {
                # "LAB01-1"
                n650 = local read "LAB01 (DISP 1)"() -> (w929:T5)
                n651 = local read "LAB01 (TEMP START)"() -> (w938:T6)
                n652 = local read "LAB01 (SETTINGS 1)"() -> (w933:T4)
                n653 = local read "LAB01-1 (SIG)"() -> (w940:T2)
                n654 = case shown="\"T-RISE TEST\"" w945 {
                  tunnel: [FALSE FALSE TRUE] -> w943
                  frame "TEST SET UP", Default {
                  }
                  frame "CYCLE TEST" {
                  }
                  frame "T-RISE TEST" {
                  }
                }
                n655 = Unbundle(w933) -> ("1 (T-RISE deg C)"=w930:dbl)  [unwired: 9 out]
                n656 = Unbundle(w938) -> ("1 (TL)"=w935:dbl, "1 (TN)"=w934:dbl)  [unwired: 2 out]
                n657 = Unbundle(w929) -> ("1 (CYCLE)"=w928:dbl)  [unwired: 5 out]
                n658 = Unbundle(w940) -> ("AMPS"=w939:dbl, "Tmp Live"=w937:dbl, "Tmp Neut"=w936:dbl)  [unwired: 2 out]
                n659 = Subtract(x=w937, y=w935) -> (x-y=w932:dbl)
                n660 = Greater?(x=w928, y=2.0) -> (0:w927:bool)
                n661 = Subtract(x=w936, y=w934) -> (x-y=w931:dbl)
                n662 = And(x=w944, y=w927) -> (x .and. y?=w941:bool)
                n663 = And(x=w943, y=w941) -> (x .and. y?=w942:bool)
                n664 = case shown="True" w942 {
                  tunnel: w939 -> [_ w961]
                  tunnel: w932 -> [_ w954]
                  tunnel: w931 -> [_ w953]
                  tunnel: w930 -> [_ w952]
                  frame False {
                  }
                  frame True {
                    # "check for amps & t-rise fail"
                    n665 = Less?(x=w961, y=5.0) -> (x < y?=w947:bool)
                    n666 = Greater?(x=w954, y=w952) -> (0:w957:bool)
                    n667 = Greater?(x=w953, y=w952) -> (0:w958:bool)
                    n668 = Or(x=w957, y=w958) -> (x .or. y?=w946:bool)
                    n669 = Select(t="AMPS LO", s=w947, f="") -> (s? t:f=w948:string)
                    n670 = Select(t="T-RISE HI", s=w946, f="") -> (s? t:f=w949:string)
                    n671 = Or(x=w947, y=w946) -> (x .or. y?=w960:bool)
                    n672 = case shown="True" w960 {
                      tunnel: w949 -> [_ w963]
                      tunnel: w948 -> [_ w962]
                      frame False {
                      }
                      frame True {
                        n673 = stacked-sequence {
                          tunnel: w963 -> [w965 _]
                          tunnel: w962 -> [w964 _]
                          frame #0 {
                            n674 = local read "LAB01-1 (TDMS)"() -> (w970:refnum<k34>)
                            n675 = Build Array(w964, w965) -> (w967:string[])
                            n676 = TDMS Write(0:w970, 5:"TEST RESULT", 7:"T-RISE FAIL ", 9:w967) -> (15:w969:errorcluster)  [unwired: 2 in, 3 out]
                            n677 = local write "data file error"(w969) -> ()
                          }
                          frame #1 {
                            n678 = local read "LAB01 (DISP 1)"() -> (w974:T5)
                            n679 = Bundle(cluster=w974, "1 (STATUS)"="STOP") -> (w973:T5)  [unwired: 5 in]
                            n680 = local write "LAB01-1 (RESULT)"(FALSE) -> ()
                            n681 = local write "LAB01 (DISP 1)"(w973) -> ()
                          }
                        }
                      }
                    }
                  }
                }
              }
            }
          }
          frame #15 {
            # "run calibration routine"
            n682 = local read "CALIBRATE"() -> (w978:bool)
            n683 = case shown="True" w978 {
              frame False {
              }
              frame True {
                n684 = stacked-sequence {
                  seq-local: [w979 _ _] -> [_ w981 _]
                  frame #0 {
                    n685 = call "CALIBRATION PASSWORD"() -> ("PASSWORD"=w979:string)  [unwired: 17 in, 2 out]
                  }
                  frame #1 {
                    n686 = Equal?(x=w981, y="7777") -> (x = y?=w980:bool)
                    n687 = case shown="True" w980 {
                      frame False {
                      }
                      frame True {
                        n688 = stacked-sequence {
                          frame #0 {
                            n689 = call "sub vi - calibration v1.vi"() -> ()  [unwired: 12 in]
                          }
                          frame #1 {
                            n690 = call "sub vi - get calibration values v1.vi"() -> ("LAB01 (CAL)"=w987:T7, "LAB02 (CAL)"=w986:T8, "LAB03 (CAL)"=w985:T7, "LAB04 (CAL)"=w984:T7, "calibration file error out"=w988:errorcluster, "LAB05 (CAL)"=w983:T7)  [unwired: 10 in]
                            n691 = local write "calibration file error out"(w988) -> ()
                            n692 = local write "LAB04 (CAL)"(w984) -> ()
                            n693 = local write "LAB05 (CAL)"(w983) -> ()
                            n694 = local write "LAB01 (CAL)"(w987) -> ()
                            n695 = local write "LAB02 (CAL)"(w986) -> ()
                            n696 = local write "LAB03 (CAL)"(w985) -> ()
                          }
                        }
                      }
                    }
                  }
                  frame #2 {
                    n697 = local write "CALIBRATE"(FALSE) -> ()
                  }
                }
              }
            }
          }
        }
        n698 = node-c288() -> ()  [unwired: 1 in, 1 out]
        "loops" <- w24
      }
      n699 = node-c288(w10) -> ()  [unwired: 1 out]
    }
  }
